vi "UV Laser Ablation and Capture.vi"() -> ()   [LabVIEW 2016]
uses:
  <vilib>/vision/NI_Vision_Development_Module.lvlib
  C:/Users/Murray group/Desktop/LabVIEW Version Controlled/UV Laser Ablation Capture Software/uc480DotNet.dll
  uc480DotNet.dll
  System.Windows.Forms
  <vilib>/Utility/miscctls.llb/LVBoundsTypeDef.ctl
  <vilib>/Utility/config.llb/NI_LVConfig.lvlib
  <vilib>/regexp/Match Regular Expression.xnode
panel:
  in  "Load ROI":bool
  in  "Save current ROI":bool
  in  "Call Last ROI":bool
  in  "Captur time\nConstant":dbl=0.001 min=0.001 step=0.001 format="%#_13g"
  out "Pre-Capture Axis 2":dbl format="%.10e"
  out "Pre-Capture Axis 1":dbl format="%.10e"
  in  "Log files":bool
  out "Axis 2 inverted?":bool
  out "Axis 1 inverted?":bool
  out "Rect height\n(px)":i32
  out "Rect width\n(px)":i32
  in  "Circle?":bool=TRUE
  out "Axis 2 group":i32
  out "Axis 1 group":i32
  in  "Microscope/Capture \nstatus button":bool=TRUE
  in  "X travel":dbl min=0.0 max=150.0 step=0.0001
  in  "Y travel":dbl min=0.0 max=150.0 step=0.0001
  in  "Laser Status":bool
  in  "SINGLE SHOT":bool
  in  "Repetition\nRate (Hz)":dbl=2.34 min=1.0 max=20.0 step=0.01 format="%.2g"
  out "Laser Com Delay":i32
  out "VISA Laser port":string
  in  "Acceleration \n(mm/s²)":dbl=20.0
  out "Camera Status":string="Load parameter"
  in  "Save configuration":bool
  in  "Stages status":bool
  in  "Transparency":u8 max=80 step=1
  in  "Overlay MSI Image":bool
  in  "Home Axes":bool
  out "Axis 2 Offset":dbl
  out "Axis 1 Offset":dbl
  out "Acceleration":dbl
  out "Velocity":dbl
  in  "Axis Initial Parameters":T1={"Velocity (units/seconds)"=1.0, "Acceleration (units/seconds²)"=20.0, "Minimum Jerk Time (seconds)"=0.005, "Maximum Jerk Time (seconds)"=0.009} {"Maximum Jerk Time (seconds)" format="%.6e"; "Minimum Jerk Time (seconds)" format="%.6e"; "Acceleration (units/seconds²)" format="%.6e"; "Velocity (units/seconds)" format="%.6e"}
  out "Axis 2":string
  out "Axis 1":string
  out "XPS_Address":string
  in  "Axes Manual Control":bool
  out "ROI Area \n(mm2)":dbl=4.035870075999999
  out "Laser on/off array":bool[][](array[boolean])
  out "Commands array":string[][](array[string])
  in  "Exit Camera":bool
  in  "Width (px)":i32=240
  in  "X offset":i32=406 step=1
  in  "Y offset":i32=693 step=1
  out "Processi time (sec)":i32=117
  in  "Processing time unit":string(combo)="sec"
  out "Process time":dbl=117.0
  in  "Mode":i32(ring) items=["RGB 32"=0, "RGB 24"=1, "Y8 Monochrom"=6]
  in  "Camera":refnum<k24>(container)
  in  "Init Camera":bool
  in  "Start Live":bool
  in  "Stop Live":bool
  in  "Load Parameter":bool
  out "Error Out":errorcluster caption="error"
  out "Bits/Pixel":i32=32
  out "Width":i32=1280
  out "Height":i32=1024
  out "Serial Number":string="4102944807"
  in  "Camera ID":i32
  in  "Zoom":dbl(ring)=1.5 items=["4X"=4.0, "2X"=2.0, "1.5X"=1.5, "1.25X"=1.25, "1X"=1.0]
  in  "Gain Boost":bool=TRUE
  in  "Snapshot":bool
  out "Output":picture
  in  "Exposure":dbl(slide)=99.80425000000001 min=0.06241666666666667 max=99.80425000000001 step=0.06241666666666667 scale=0.06241666666666667..99.80425000000001 scale format="%#.3g"
  in  "Framerate":dbl(slide)=10.002522802986672 min=0.47411700449083627 max=15.001275108384213 step=0.014032998230481021 scale=0.47411700449083627..15.001275108384213 scale format="%#.3g"
  in  "Pixelclock":i32(slide)=24 min=5 max=40 step=1 scale=5.0..40.0
  in  "error in (no error)":errorcluster
  out "error out":errorcluster
  in  "Precision (%)":dbl=1.0 min=1.0 max=100.0 step=1.0 format="%#_3g"
  in  "Process Image":bool
  in  "Pixel size":dbl=12.19 step=0.01
  in  "Speed (µm/s)":i32=1000
  in  "Heigth (px)":i32=240
  in  "Height \nstep divider":i32=2
  out "Rect height\n(µm/px)":i32=2267
  out "Rect. width \n(µm/px))":i32=2267
  out "Source":T2(plugin-control)
  in  "Open \nManual":bool
  in  "Capture":bool
  out "Log":string
  out "Laser Operation":bool
  in  "LASER":bool
  in  "LAMP":bool
  in  "EXIT":bool
  # "Laser Control"
  # "Stages Control"
  # "Camera Control"
  # "ROI Processing"
  # "Laser spot size and position"
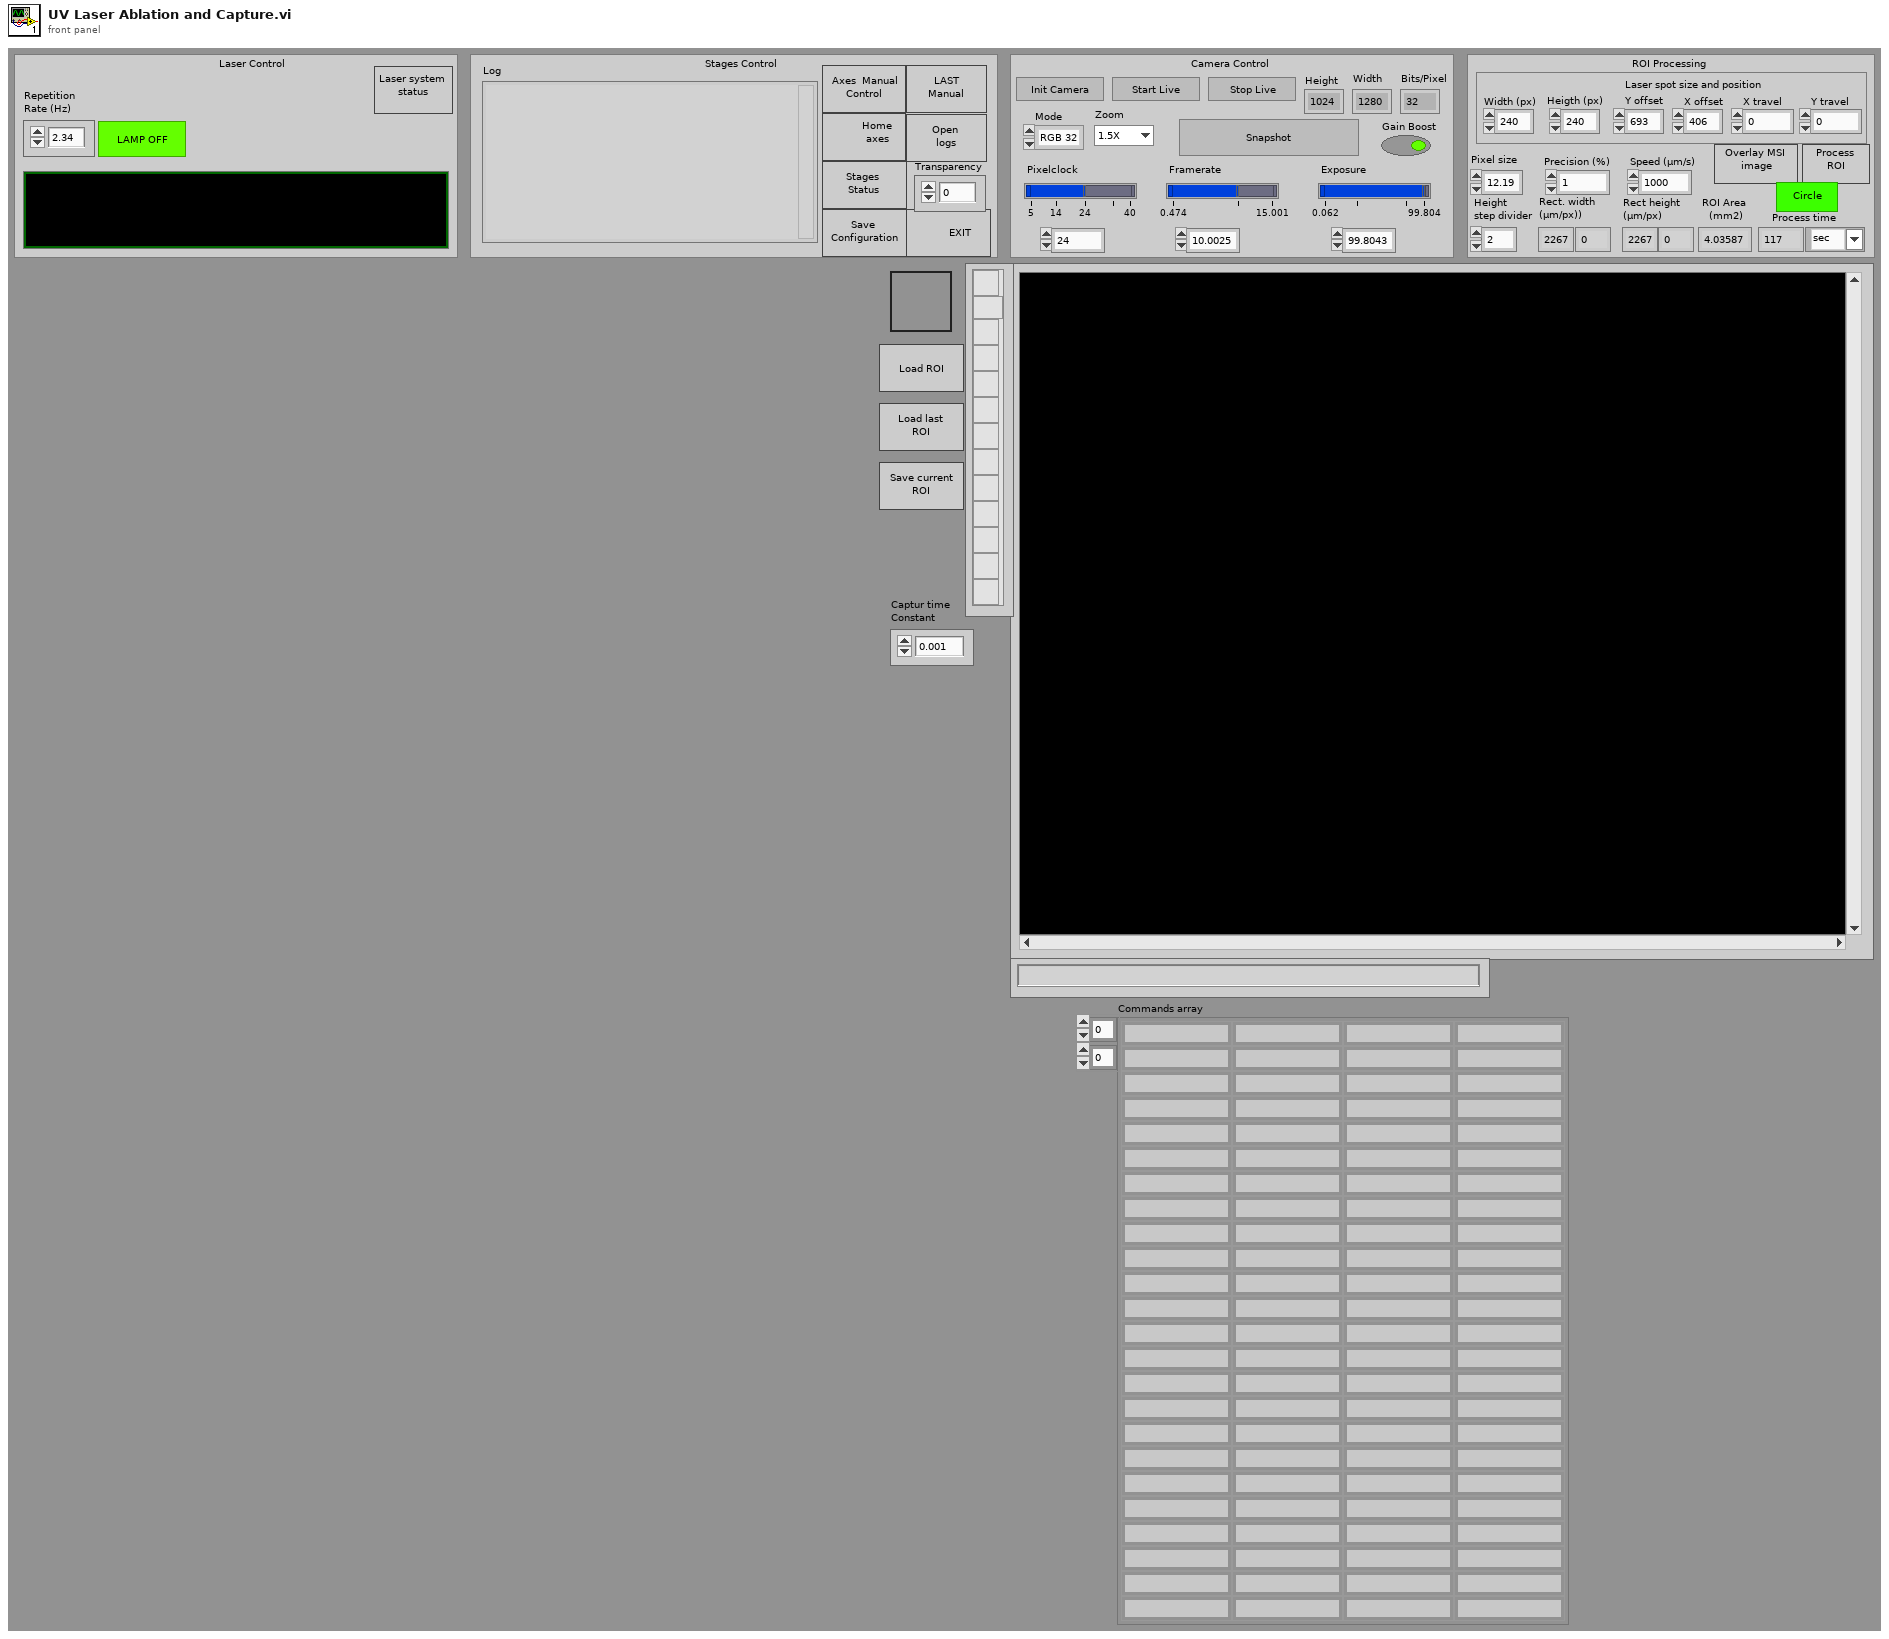
[diagram p1: front panel]
types:
  T1 = cluster{"Velocity (units/seconds)":dbl, "Acceleration (units/seconds²)":dbl, "Minimum Jerk Time (seconds)":dbl, "Maximum Jerk Time (seconds)":dbl}
  T2 = typedef "IMAQ Image.ctl" = refnum<image>
  T3 = typedef "LVBoundsTypeDef.ctl" = cluster{"Width":u32, "Height":u32}
  T4 = enum8{"Enabled", "Disabled", "Disabled and Grayed Out"}
  T5 = typedef "NI_LVConfig.lvlib/Config Data RefNum.ctl" = refnum<k1>
  T6 = enum16{"open", "replace", "create", "open or create", "replace or create", "replace or create with confirmation"}
  T7 = enum32{"Invalid", "Standard", "Closed", "Hidden", "Minimized", "Maximized"}
  T8 = enum32{"invalid app kind", "Development System", "Run Time System", "Student Edition", "Embedded LabVIEW", "Evaluation", "Custom"}
  T9 = cluster{"connection TCP":refnum<k5>, "LogTo File":bool, "Log File refnum":refnum<file>, "no error if error log":bool}
  T10 = typedef "Image Type" = u32
  T11 = cluster{"Global Rectangle":i32[], "Contours":cluster{"Contour Type":u32, "ROI Type":u32, "Points":i32[]}[]}
  T12 = cluster{"Global Rectangle[0]":i32, "Global Rectangle[1]":i32}
  T13 = typedef "ROI Descriptor" = cluster{"Global Rectangle":i32[], "Contours":cluster{"ID":enum32{"External", "Internal"}, "Type":u32, "Coordinates":i32[]}[]}
  T14 = cluster{"ID":enum32{"External", "Internal"}, "Type":u32, "Coordinates":i32[]}[]
  T15 = cluster{"ID":enum32{"External", "Internal"}, "Type":u32, "Coordinates":i32[]}
  T16 = cluster{"Contour Type":u32, "ROI Type":u32, "Points":i32[]}[]
  T17 = cluster{"Contour Type":u32, "ROI Type":u32, "Points":i32[]}
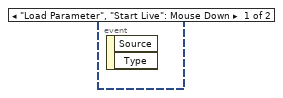
[diagram p2: hidden frame]
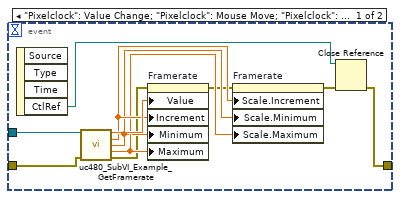
[diagram p3: hidden frame]
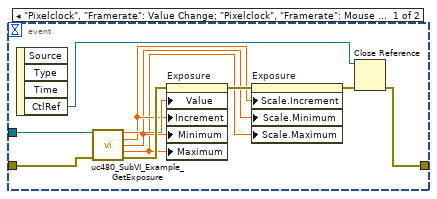
[diagram p4: hidden frame]
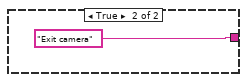
[diagram p5: hidden frame]
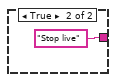
[diagram p6: hidden frame]
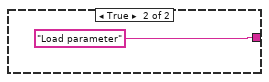
[diagram p7: hidden frame]
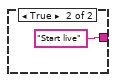
[diagram p8: hidden frame]
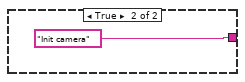
[diagram p9: hidden frame]
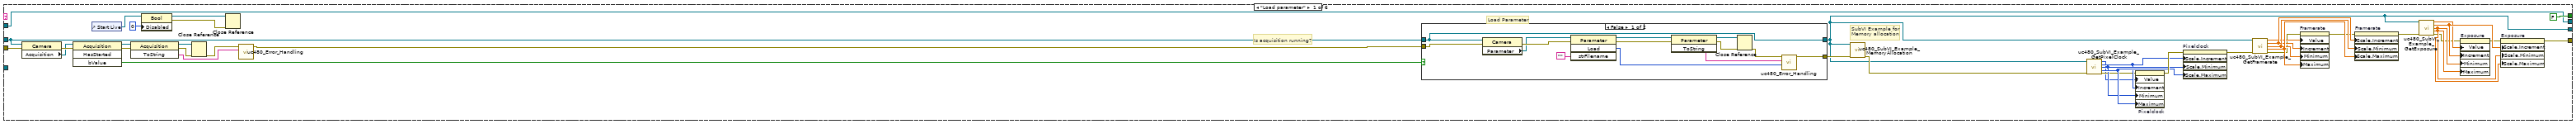
[diagram p10: hidden frame]
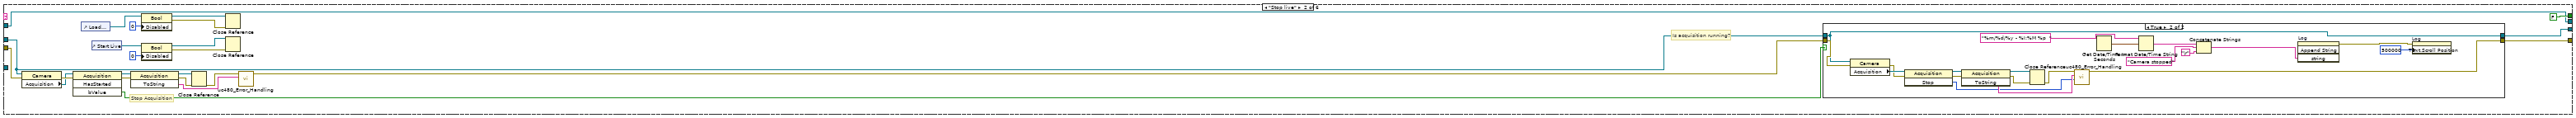
[diagram p12: hidden frame]
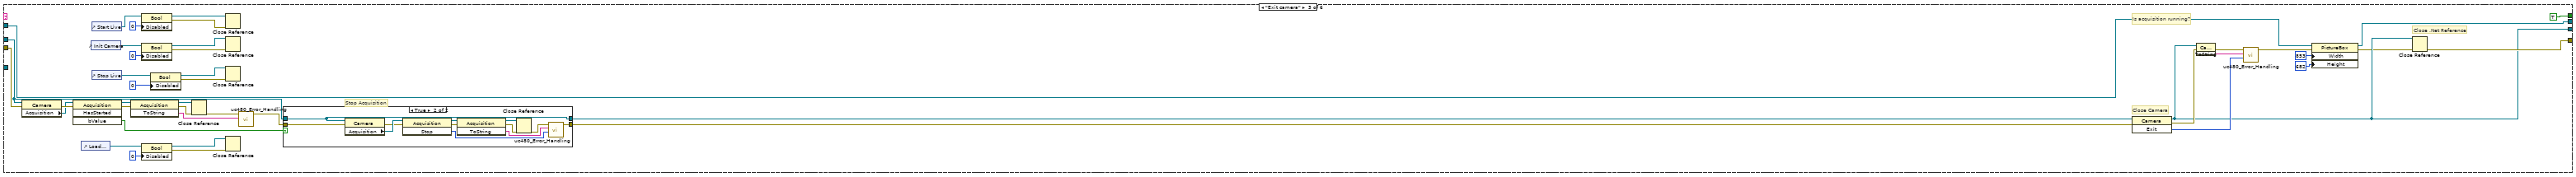
[diagram p14: hidden frame]
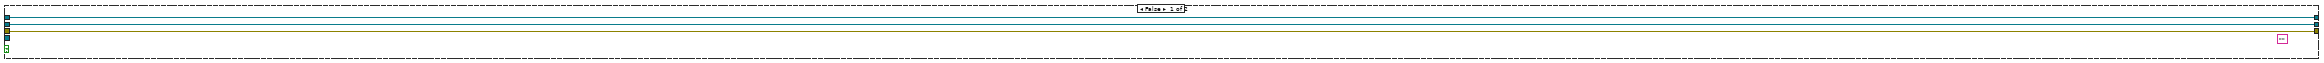
[diagram p16: hidden frame]
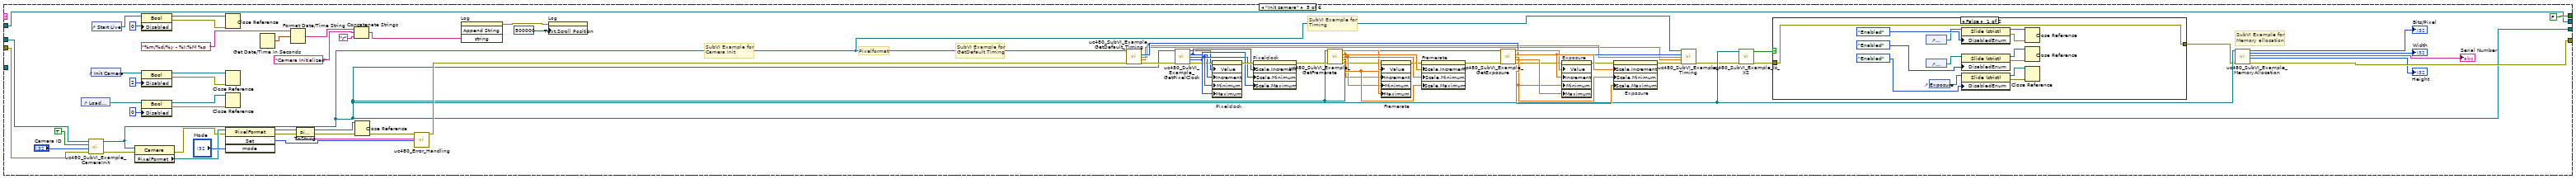
[diagram p18: hidden frame]
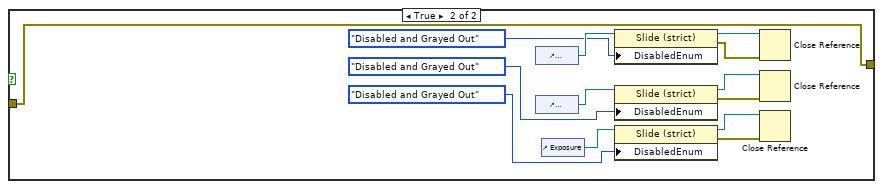
[diagram p19: hidden frame]
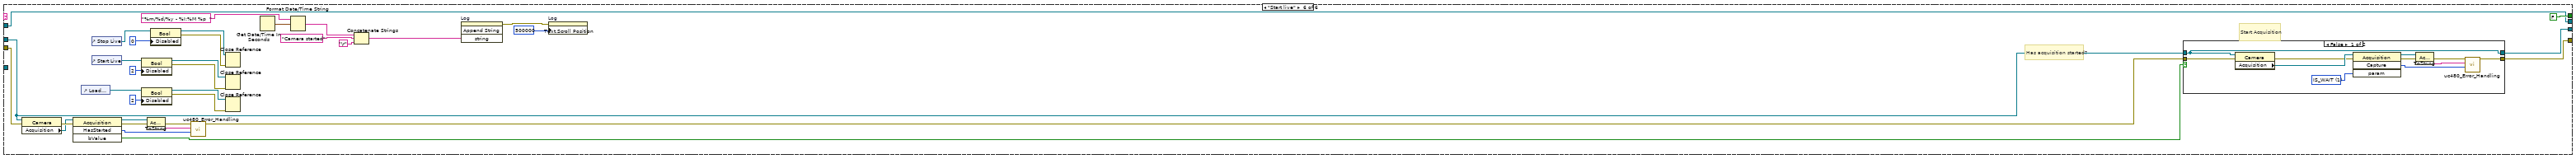
[diagram p20: hidden frame]
diagram:
  w65 = 1 items=["None", "FixedSingle", "Fixed3D"] ("BorderStyle")
  # "Button and controls"
  # "Camera control buttons"
  n1 = property class="PictureBox"(reference="Camera", "BorderStyle"=w65, "Width"=853, "Height"=682) -> (reference out=w53:refnum<k24>, error out=w54:errorcluster)  [unwired: 1 in]
  n2 = property class="PictureBox"(reference=w53, error in=w54) -> (reference out=w52:refnum<k24>, error out=w51:errorcluster, "Handle"=w50:refnum<k24>)
  n3 = while "Camera Control" {
    shift-right: [w82] -> _
    shift-left: w51 -> [w88]
    shift-right: [w85] -> _
    shift-left: _ -> [w78]
    shift-right: [w80] -> _
    shift-left: w52 -> [w81]
    tunnel: w50 -> [w79]
    stop <- w86 stop-if-true
    # ".NetReference"
    # ".Net Reference"
    n4 = event shown="[1] Timeout" {
      selector: _ -> [_ _]
      dyn-events: _ -> [_ _]
      timeout: 0 -> [_ _]
      event "Load Parameter", "Start Live": Mouse Down {
        n5 = event-data() -> ()  [unwired: 1 in, 2 out]
      }
      event Timeout {
        n6 = event-data() -> ()  [unwired: 1 in, 2 out]
      }
    }
    n7 = event shown="[1] Timeout" {
      selector: _ -> [_ _]
      dyn-events: _ -> [_ _]
      timeout: 0 -> [_ _]
      tunnel: [w102 w113] -> w89
      tunnel: w88 -> [w112 w113]
      tunnel: w78 -> [w111 _]
      event "Pixelclock": Value Change; "Pixelclock": Mouse Move; "Pixelclock": Key Down; "Pixelclock": Mouse Up {
        n8 = event-data() -> ("CtlRef"=w104:refnum<vi>)  [unwired: 1 in, 3 out]
        n9 = call "uc480_SubVI_Example_GetFramerate.vi"(".NET (Reference)"=w111, "Error In"=w112) -> ("Framerate"=w110:dbl, "Inc"=w109:dbl, "Min"=w107:dbl, "Max"=w108:dbl, "error out"=w106:errorcluster)  [unwired: 9 in]
        n10 = property on="Framerate" class="Slide (strict)"(error in=w106, "Value"=w110, "Increment"=w109, "Minimum"=w107, "Maximum"=w108) -> (error out=w105:errorcluster)  [unwired: 1 in, 1 out]
        n11 = property on="Framerate" class="Slide (strict)"(error in=w105, "Scale.Increment"=w109, "Scale.Minimum"=w107, "Scale.Maximum"=w108) -> (error out=w103:errorcluster)  [unwired: 1 in, 1 out]
        n12 = Close Reference(reference=w104, error in (no error)=w103) -> (error out=w102:errorcluster)
      }
      event Timeout {
        n13 = event-data() -> ()  [unwired: 1 in, 2 out]
      }
    }
    n14 = case shown="False" "Load Parameter" {
      tunnel: ["" "Load parameter"] -> w95
      frame False {
      }
      frame True {
      }
    }
    n15 = case shown="False" "Init Camera" {
      tunnel: ["" "Init camera"] -> w99
      frame False {
      }
      frame True {
      }
    }
    n16 = case shown="False" "Exit Camera" {
      tunnel: ["" "Exit camera"] -> w93
      frame False {
      }
      frame True {
      }
    }
    n17 = event shown="[1] Timeout" {
      selector: _ -> [_ _]
      dyn-events: _ -> [_ _]
      timeout: 0 -> [_ _]
      tunnel: w89 -> [w124 w125]
      tunnel: [w114 w125] -> w91
      tunnel: w78 -> [w123 _]
      event "Pixelclock", "Framerate": Value Change; "Pixelclock", "Framerate": Mouse Move; "Pixelclock", "Framerate": Key Down; "Pixelclock", "Framerate": Mouse Up {
        n18 = event-data() -> ("CtlRef"=w116:refnum<vi>)  [unwired: 1 in, 3 out]
        n19 = call "uc480_SubVI_Example_GetExposure.vi"(".NET (Reference)"=w123, "Error In"=w124) -> ("Exposure"=w120:dbl, "Inc"=w119:dbl, "Min"=w118:dbl, "Max"=w117:dbl, "Error out"=w121:errorcluster)  [unwired: 9 in]
        n20 = property on="Exposure" class="Slide (strict)"(error in=w121, "Value"=w120, "Increment"=w119, "Minimum"=w118, "Maximum"=w117) -> (error out=w122:errorcluster)  [unwired: 1 in, 1 out]
        n21 = property on="Exposure" class="Slide (strict)"(error in=w122, "Scale.Increment"=w119, "Scale.Minimum"=w118, "Scale.Maximum"=w117) -> (error out=w115:errorcluster)  [unwired: 1 in, 1 out]
        n22 = Close Reference(reference=w116, error in (no error)=w115) -> (error out=w114:errorcluster)
      }
      event Timeout {
        n23 = event-data() -> ()  [unwired: 1 in, 2 out]
      }
    }
    n24 = case shown="False" "Start Live" {
      tunnel: ["" "Start live"] -> w98
      frame False {
      }
      frame True {
      }
    }
    n25 = case shown="False" "Stop Live" {
      tunnel: ["" "Stop live"] -> w94
      frame False {
      }
      frame True {
      }
    }
    n26 = local read "Camera Status"() -> (w75:string)
    n27 = Concatenate Strings(w99, w98, w95, w94, w93) -> (→"Camera Status":string)
    n28 = case shown="Default" w75 {
      tunnel: w78 -> [w168 w208 w266 w308 w488 w547]
      tunnel: w91 -> [w171 w209 w267 w318 w487 w548]
      tunnel: [w142 w207 w275 w317 w446 w546] -> w85
      tunnel: [w143 w206 w276 w316 w483 w544] -> w84
      tunnel: [FALSE FALSE TRUE FALSE FALSE FALSE] -> w86
      tunnel: w81 -> [w141 w200 w248 w300 w441 w537]
      tunnel: [w141 w200 w247 w299 w441 w537] -> w80
      tunnel: w79 -> [_ _ _ w296 _ _]
      frame "Load parameter" {
        # "SubVI Example for \nMemory allocation"
        # "Is acquisition running?"
        # "Load Parameter"
        n29 = property class="Camera"(reference=w168, error in=w171) -> (error out=w176:errorcluster, "Acquisition"=w175:refnum<k24>)  [unwired: 1 out]
        n30 = invoke class="Acquisition" method="HasStarted"(reference=w175, error in=w176) -> (reference out=w172:refnum<k24>, error out=w174:errorcluster, "bValue"=w170:bool)  [unwired: 2 in, 1 out]
        n31 = control-ref of="Start Live"() -> (w166:refnum<vi>)
        n32 = invoke class="Acquisition" method="ToString"(reference=w172, error in=w174) -> (reference out=w138:refnum<k24>, error out=w137:errorcluster, "ToString"=w173:string)  [unwired: 1 in]
        n33 = property class="Bool"(reference=w166, "Disabled"=u8 0 ("Deaktiviert")) -> (reference out=w140:refnum<vi>, error out=w139:errorcluster)  [unwired: 1 in]
        n34 = Close Reference(reference=w138, error in (no error)=w137) -> (error out=w136:errorcluster)
        n35 = Close Reference(reference=w140, error in (no error)=w139) -> ()  [unwired: 1 out]
        n36 = call "uc480_Error_Handling.vi"("Error String"=w173, "Error In"=w136) -> ("Error Out"=w169:errorcluster)  [unwired: 9 in]
        n37 = case shown="False" w170 {
          tunnel: w169 -> [w184 w191]
          tunnel: w168 -> [w182 w192]
          tunnel: [w183 w191] -> w167
          tunnel: [w182 w192] -> w142
          frame False {
            n38 = property class="Camera"(reference=w182, error in=w184) -> (error out=w186:errorcluster, "Parameter"=w185:refnum<k24>)  [unwired: 1 out]
            n39 = invoke class="Parameter" method="Load"(reference=w185, error in=w186, "strFilename"="") -> (reference out=w188:refnum<k24>, error out=w189:errorcluster, "Load"=w181:i32)  [unwired: 1 in, 1 out]
            n40 = invoke class="Parameter" method="ToString"(reference=w188, error in=w189) -> (reference out=w178:refnum<k24>, error out=w180:errorcluster, "ToString"=w190:string)  [unwired: 1 in]
            n41 = Close Reference(reference=w178, error in (no error)=w180) -> (error out=w179:errorcluster)
            n42 = call "uc480_Error_Handling.vi"("Error Code"=w181, "Error String"=w190, "Error In"=w179) -> ("Error Out"=w183:errorcluster)  [unwired: 8 in]
          }
          frame True {
          }
        }
        n43 = call "uc480_SubVI_Example_MemoryAllocation.vi"(".NET (Reference)"=w142, "Error In"=w167) -> ("Error Out"=w144:errorcluster)  [unwired: 13 in, 4 out]
        n44 = call "uc480_SubVI_Example_GetPixelClock.vi"(".NET (Reference)"=w142, "Error In"=w144) -> ("Pixel Clock"=w145:i32, "Inc"=w147:i32, "Min"=w148:i32, "Max"=w149:i32, "error out"=w146:errorcluster)  [unwired: 9 in]
        n45 = property on="Pixelclock" class="Slide (strict)"(error in=w146, "Value"=w145, "Increment"=w147, "Minimum"=w148, "Maximum"=w149) -> (error out=w150:errorcluster)  [unwired: 1 in, 1 out]
        n46 = property on="Pixelclock" class="Slide (strict)"(error in=w150, "Scale.Increment"=w147, "Scale.Minimum"=w148, "Scale.Maximum"=w149) -> (error out=w151:errorcluster)  [unwired: 1 in, 1 out]
        n47 = call "uc480_SubVI_Example_GetFramerate.vi"(".NET (Reference)"=w142, "Error In"=w151) -> ("Framerate"=w154:dbl, "Inc"=w155:dbl, "Min"=w156:dbl, "Max"=w157:dbl, "error out"=w153:errorcluster)  [unwired: 9 in]
        n48 = property on="Framerate" class="Slide (strict)"(error in=w153, "Value"=w154, "Increment"=w155, "Minimum"=w156, "Maximum"=w157) -> (error out=w152:errorcluster)  [unwired: 1 in, 1 out]
        n49 = property on="Framerate" class="Slide (strict)"(error in=w152, "Scale.Increment"=w155, "Scale.Minimum"=w156, "Scale.Maximum"=w157) -> (error out=w158:errorcluster)  [unwired: 1 in, 1 out]
        n50 = call "uc480_SubVI_Example_GetExposure.vi"(".NET (Reference)"=w142, "Error In"=w158) -> ("Exposure"=w161:dbl, "Inc"=w162:dbl, "Min"=w163:dbl, "Max"=w164:dbl, "Error out"=w159:errorcluster)  [unwired: 9 in]
        n51 = property on="Exposure" class="Slide (strict)"(error in=w159, "Value"=w161, "Increment"=w162, "Minimum"=w163, "Maximum"=w164) -> (error out=w160:errorcluster)  [unwired: 1 in, 1 out]
        n52 = property on="Exposure" class="Slide (strict)"(error in=w160, "Scale.Increment"=w162, "Scale.Minimum"=w163, "Scale.Maximum"=w164) -> (error out=w143:errorcluster)  [unwired: 1 in, 1 out]
      }
      frame "Stop live" {
        # "Is acquisition running?"
        # "Stop Acquisition"
        n53 = property class="Camera"(reference=w208, error in=w209) -> (error out=w216:errorcluster, "Acquisition"=w215:refnum<k24>)  [unwired: 1 out]
        n54 = invoke class="Acquisition" method="HasStarted"(reference=w215, error in=w216) -> (reference out=w210:refnum<k24>, error out=w212:errorcluster, "bValue"=w214:bool)  [unwired: 2 in, 1 out]
        n55 = control-ref of="Load Parameter"() -> (w204:refnum<vi>)
        n56 = control-ref of="Start Live"() -> (w201:refnum<vi>)
        n57 = invoke class="Acquisition" method="ToString"(reference=w210, error in=w212) -> (reference out=w193:refnum<k24>, error out=w195:errorcluster, "ToString"=w211:string)  [unwired: 1 in]
        n58 = property class="Bool"(reference=w204, "Disabled"=u8 0 ("Deaktiviert")) -> (reference out=w199:refnum<vi>, error out=w198:errorcluster)  [unwired: 1 in]
        n59 = property class="Bool"(reference=w201, "Disabled"=u8 0 ("Deaktiviert")) -> (reference out=w197:refnum<vi>, error out=w196:errorcluster)  [unwired: 1 in]
        n60 = Close Reference(reference=w193, error in (no error)=w195) -> (error out=w194:errorcluster)
        n61 = Close Reference(reference=w199, error in (no error)=w198) -> ()  [unwired: 1 out]
        n62 = Close Reference(reference=w197, error in (no error)=w196) -> ()  [unwired: 1 out]
        n63 = call "uc480_Error_Handling.vi"("Error String"=w211, "Error In"=w194) -> ("Error Out"=w213:errorcluster)  [unwired: 9 in]
        n64 = case shown="True" w214 {
          tunnel: [w218 w237] -> w206
          tunnel: w213 -> [w218 w238]
          tunnel: w208 -> [w217 w230]
          tunnel: [w217 w230] -> w207
          frame False {
          }
          frame True {
            n65 = property class="Camera"(reference=w230, error in=w238) -> (error out=w234:errorcluster, "Acquisition"=w235:refnum<k24>)  [unwired: 1 out]
            n66 = invoke class="Acquisition" method="Stop"(reference=w235, error in=w234) -> (reference out=w232:refnum<k24>, error out=w233:errorcluster, "Stop"=w231:i32)  [unwired: 1 in]
            n67 = invoke class="Acquisition" method="ToString"(reference=w232, error in=w233) -> (reference out=w227:refnum<k24>, error out=w229:errorcluster, "ToString"=w236:string)  [unwired: 1 in]
            n68 = Close Reference(reference=w227, error in (no error)=w229) -> (error out=w228:errorcluster)
            n69 = call "uc480_Error_Handling.vi"("Error Code"=w231, "Error String"=w236, "Error In"=w228) -> ("Error Out"=w237:errorcluster)  [unwired: 8 in]
            n70 = Get Date/Time In Seconds() -> (seconds since 1Jan1904=w225:timestamp)
            n71 = Format Date/Time String(time format string (%c)="%m/%d/%y - %I:%M %p  ", seconds (now)=w225) -> (date/time string=w226:string)  [unwired: 1 in]
            n72 = Concatenate Strings(w226, "Camera stopped", "\r") -> (w221:string)
            n73 = invoke on="Log" class="Str" method="Append String"("string"=w221) -> (error out=w219:errorcluster)  [unwired: 3 in, 3 out]
            n74 = property on="Log" class="Str"(error in=w219, "Text.Scroll Position"=u32 500000) -> ()  [unwired: 1 in, 2 out]
          }
        }
      }
      frame "Exit camera" {
        # "Close .Net Reference"
        # "Is acquisition running?"
        # "Stop Acquisition"
        # "Close Camera"
        n75 = property class="Camera"(reference=w266, error in=w267) -> (error out=w274:errorcluster, "Acquisition"=w273:refnum<k24>)  [unwired: 1 out]
        n76 = invoke class="Acquisition" method="HasStarted"(reference=w273, error in=w274) -> (reference out=w268:refnum<k24>, error out=w270:errorcluster, "bValue"=w272:bool)  [unwired: 2 in, 1 out]
        n77 = control-ref of="Load Parameter"() -> (w257:refnum<vi>)
        n78 = control-ref of="Init Camera"() -> (w259:refnum<vi>)
        n79 = control-ref of="Start Live"() -> (w258:refnum<vi>)
        n80 = control-ref of="Stop Live"() -> (w256:refnum<vi>)
        n81 = invoke class="Acquisition" method="ToString"(reference=w268, error in=w270) -> (reference out=w253:refnum<k24>, error out=w255:errorcluster, "ToString"=w269:string)  [unwired: 1 in]
        n82 = property class="Bool"(reference=w258, "Disabled"=u8 0 ("Deaktiviert")) -> (reference out=w242:refnum<vi>, error out=w241:errorcluster)  [unwired: 1 in]
        n83 = property class="Bool"(reference=w259, "Disabled"=u8 0 ("Deaktiviert")) -> (reference out=w240:refnum<vi>, error out=w239:errorcluster)  [unwired: 1 in]
        n84 = property class="Bool"(reference=w257, "Disabled"=u8 0 ("Deaktiviert")) -> (reference out=w244:refnum<vi>, error out=w243:errorcluster)  [unwired: 1 in]
        n85 = property class="Bool"(reference=w256, "Disabled"=u8 0 ("Deaktiviert")) -> (reference out=w246:refnum<vi>, error out=w245:errorcluster)  [unwired: 1 in]
        n86 = Close Reference ("Close Referenz")(reference=w253, error in (no error)=w255) -> (error out=w254:errorcluster)
        n87 = Close Reference(reference=w242, error in (no error)=w241) -> ()  [unwired: 1 out]
        n88 = Close Reference(reference=w240, error in (no error)=w239) -> ()  [unwired: 1 out]
        n89 = Close Reference(reference=w246, error in (no error)=w245) -> ()  [unwired: 1 out]
        n90 = Close Reference(reference=w244, error in (no error)=w243) -> ()  [unwired: 1 out]
        n91 = call "uc480_Error_Handling.vi"("Error String"=w269, "Error In"=w254) -> ("Error Out"=w271:errorcluster)  [unwired: 9 in]
        n92 = case shown="True" w272 {
          tunnel: [w283 w294] -> w264
          tunnel: w271 -> [w283 w295]
          tunnel: w266 -> [w282 w287]
          tunnel: [w282 w287] -> w265
          frame False {
          }
          frame True {
            n93 = property class="Camera"(reference=w287, error in=w295) -> (error out=w291:errorcluster, "Acquisition"=w292:refnum<k24>)  [unwired: 1 out]
            n94 = invoke class="Acquisition" method="Stop"(reference=w292, error in=w291) -> (reference out=w289:refnum<k24>, error out=w290:errorcluster, "Stop"=w288:i32)  [unwired: 1 in]
            n95 = invoke class="Acquisition" method="ToString"(reference=w289, error in=w290) -> (reference out=w284:refnum<k24>, error out=w286:errorcluster, "ToString"=w293:string)  [unwired: 1 in]
            n96 = Close Reference ("Close Referenz")(reference=w284, error in (no error)=w286) -> (error out=w285:errorcluster)
            n97 = call "uc480_Error_Handling.vi"("Error Code"=w288, "Error String"=w293, "Error In"=w285) -> ("Error Out"=w294:errorcluster)  [unwired: 8 in]
          }
        }
        n98 = invoke class="Camera" method="Exit"(reference=w265, error in=w264) -> (reference out=w275:refnum<k24>, error out=w278:errorcluster, "Exit"=w277:i32)  [unwired: 1 in]
        n99 = invoke class="Camera" method="ToString"(reference=w275, error in=w278) -> (error out=w279:errorcluster, "ToString"=w280:string)  [unwired: 1 in, 1 out]
        n100 = call "uc480_Error_Handling.vi"("Error Code"=w277, "Error String"=w280, "Error In"=w279) -> ("Error Out"=w252:errorcluster)  [unwired: 8 in]
        n101 = property class="PictureBox"(reference=w248, error in=w252, "Width"=853, "Height"=682) -> (reference out=w247:refnum<k24>, error out=w251:errorcluster)
        n102 = Close Reference ("Close Referenz")(reference=w275, error in (no error)=w251) -> (error out=w276:errorcluster)
      }
      frame Default {
        # "SubVI Example for Timing"
        # "Has acquisition started?"
        n103 = call "uc480_SubVI_Example_Timing.vi"(".NET (Reference)"=w308, "Pixelclock"="Pixelclock", "Exposure time"="Exposure", "Framerate"="Framerate", "Error In"=w318) -> ("Pixelclock"=w311:i32, "Exposure time"=w310:dbl, "Framerate"=w309:dbl, "Error Out"=w315:errorcluster)  [unwired: 7 in]
        n104 = property on="Framerate" class="Schieber (strikt)"(error in=w315, "Scale.RngStart"=w309) -> (error out=w314:errorcluster)  [unwired: 1 in, 1 out]
        n105 = property on="Exposure" class="Schieber (strikt)"(error in=w314, "Scale.RngStart"=w310) -> (error out=w313:errorcluster)  [unwired: 1 in, 1 out]
        n106 = property on="Pixelclock" class="Schieber (strikt)"(error in=w313, "Scale.RngStart"=w311) -> (error out=w312:errorcluster)  [unwired: 1 in, 1 out]
        n107 = property class="Camera"(reference=w308, error in=w312) -> (reference out=w301:refnum<k24>, error out=w324:errorcluster, "Acquisition"=w323:refnum<k24>)
        n108 = invoke class="Acquisition" method="HasStarted"(reference=w323, error in=w324) -> (reference out=w298:refnum<k24>, error out=w320:errorcluster, "HasStarted"=w319:i32, "bValue"=w297:bool)  [unwired: 2 in]
        n109 = invoke class="Acquisition" method="ToString"(reference=w298, error in=w320) -> (reference out=w302:refnum<k24>, error out=w322:errorcluster, "ToString"=w321:string)  [unwired: 1 in]
        n110 = call "uc480_Error_Handling.vi"("Error Code"=w319, "Error String"=w321, "Error In"=w322) -> ("Error Out"=w304:errorcluster)  [unwired: 8 in]
        n111 = Close Reference(reference=w302, error in (no error)=w304) -> (error out=w303:errorcluster)
        n112 = case "Show Image" shown="True" w297 {
          tunnel: [w328 w340] -> w316
          tunnel: w303 -> [w328 w368]
          tunnel: w301 -> [w327 w332]
          tunnel: [w327 w336] -> w317
          tunnel: w300 -> [w326 w357]
          tunnel: [w326 w334] -> w299
          tunnel: w296 -> [_ w364]
          frame False {
            (unwired) ""
          }
          frame True {
            n113 = local read "Height"() -> (w361:i32)
            n114 = local read "Width"() -> (w362:i32)
            n115 = Quotient & Remainder(x=w362, y="Zoom") -> (floor(x/y)=w359:dbl)  [unwired: 1 out]
            n116 = Quotient & Remainder(x=w361, y="Zoom") -> (floor(x/y)=w358:dbl)  [unwired: 1 out]
            n117 = To Long Integer(number=w359) -> (32bit integer=w331:i32)
            n118 = To Long Integer(number=w358) -> (32bit integer=w330:i32)
            n119 = property class="PictureBox"(reference=w357, error in=w368, "Width"=w331, "Height"=w330) -> (reference out=w334:refnum<k24>, error out=w363:errorcluster)
            n120 = property class="Camera"(reference=w332, error in=w363) -> (reference out=w333:refnum<k24>, error out=w370:errorcluster, "Memory"=w371:refnum<k24>)
            n121 = invoke class="Memory" method="GetActive"(reference=w371, error in=w370) -> (reference out=w365:refnum<k24>, error out=w366:errorcluster, "s32MemId"=w337:i32)  [unwired: 2 in, 1 out]
            n122 = property class="Camera"(reference=w333, error in=w366) -> (reference out=w345:refnum<k24>, error out=w369:errorcluster, "Display"=w354:refnum<k24>)
            n123 = invoke class="Display" method="Render"(reference=w354, error in=w369, "memID"=w337, "windowHandle"=w364) -> (reference out=w355:refnum<k24>, error out=w356:errorcluster)  [unwired: 1 in, 3 out]
            n124 = property class="Camera"(reference=w345, error in=w356) -> (reference out=w336:refnum<k24>, error out=w352:errorcluster, "Gain"=w350:refnum<k24>)
            n125 = property class="Gain"(reference=w350, error in=w352) -> (reference out=w351:refnum<k24>, error out=w347:errorcluster, "Hardware"=w346:refnum<k24>)
            n126 = property class="GainHardware"(reference=w346, error in=w347) -> (reference out=w343:refnum<k24>, error out=w348:errorcluster, "Boost"=w349:refnum<k24>)
            n127 = property class="GainBoost"(reference=w349, error in=w348, "Enabled"="Gain Boost") -> (reference out=w344:refnum<k24>, error out=w335:errorcluster)
            n128 = case "Snapshot control" shown="True" "Snapshot" {
              tunnel: w332 -> [_ w392]
              tunnel: w335 -> [w372 w396]
              tunnel: [w372 w383] -> w329
              tunnel: w331 -> [_ w386]
              tunnel: w330 -> [_ w385]
              frame False {
              }
              frame True {
                n129 = property class="Camera"(reference=w392, error in=w396) -> (error out=w416:errorcluster, "Memory"=w415:refnum<k24>)  [unwired: 1 out]
                n130 = local read "Zoom"() -> (w391:dbl)
                n131 = invoke class="Memory" method="GetList"(reference=w415, error in=w416) -> (reference out=w421:refnum<k24>, error out=w420:errorcluster, "GetList"=w422:i32, "idList"=w409:i32[])  [unwired: 2 in]
                n132 = Bundle(cluster=T3 {"Width"=0, "Height"=0} ("Draw Area Size"), "Width"=w386, "Height"=w385) -> (w387:T3)
                n133 = Divide(x=1.0, y=w391) -> (x/y=w389:dbl)
                n134 = property on="Output" class="Pict"("ZoomFactor"=w389, "Draw Area Size"=w387) -> ()  [unwired: 2 in, 2 out]
                n135 = invoke class="Memory" method="ToString"(reference=w421, error in=w420) -> (reference out=w394:refnum<k24>, error out=w404:errorcluster, "ToString"=w419:string)  [unwired: 1 in]
                n136 = Index Array(array=w409, index=0 ("Active \nAcquisition Buffer")) -> (element=w406:i32)
                n137 = Index Array(array=w409, index=u32 0 ("Active \nOutput Buffer")) -> (element=w405:i32)
                n138 = Close Reference(reference=w394, error in (no error)=w404) -> (error out=w403:errorcluster)
                n139 = call "uc480_Error_Handling.vi"("Error Code"=w422, "Error String"=w419, "Error In"=w403) -> ("Error Out"=w412:errorcluster)  [unwired: 8 in]
                n140 = Get Date/Time In Seconds() -> (seconds since 1Jan1904=w376:timestamp)
                n141 = property class="Camera"(reference=w392, error in=w412) -> (error out=w411:errorcluster, "Memory"=w410:refnum<k24>)  [unwired: 1 out]
                n142 = Format Date/Time String(time format string (%c)="%m/%d/%y -%I:%M %p  ", seconds (now)=w376) -> (date/time string=w375:string)  [unwired: 1 in]
                n143 = invoke class="Memory" method="SetActive"(reference=w410, error in=w411, "s32MemId"=w406) -> (reference out=w395:refnum<k24>, error out=w402:errorcluster)  [unwired: 1 in, 2 out]
                n144 = Concatenate Strings(w375, "Snapshot taken", "\r") -> (w380:string)
                n145 = Close Reference(reference=w395, error in (no error)=w402) -> (error out=w401:errorcluster)
                n146 = invoke on="Log" class="Str" method="Append String"("string"=w380) -> (error out=w373:errorcluster)  [unwired: 3 in, 3 out]
                n147 = property class="Camera"(reference=w392, error in=w401) -> (error out=w418:errorcluster, "Memory"=w407:refnum<k24>)  [unwired: 1 out]
                n148 = invoke class="Memory" method="CopyToArray"(reference=w407, error in=w418, "s32MemId"=w405) -> (reference out=w397:refnum<k24>, error out=w398:errorcluster, "u8Image"=w417:u8[])  [unwired: 2 in, 2 out]
                n149 = property on="Log" class="Str"(error in=w373, "Text.Scroll Position"=u32 500000) -> ()  [unwired: 1 in, 2 out]
                n150 = invoke class="Memory" method="ToString"(reference=w397, error in=w398) -> (reference out=w393:refnum<k24>, error out=w400:errorcluster, "ToString"=w423:string)  [unwired: 1 in]
                n151 = Close Reference(reference=w393, error in (no error)=w400) -> (error out=w399:errorcluster)
                n152 = call "uc480_Error_Handling.vi"("Error String"=w423, "Error In"=w399) -> ("Error Out"=w414:errorcluster)  [unwired: 9 in]
                n153 = call "uc480_ArrayToImage.vi"("Error In"=w414, "InArray"=w417, ".NET (Reference)"=w392) -> ("Error Out"=w382:errorcluster, "Image"=w384:picture)  [unwired: 7 in]
                "Output" <- w384
                n154 = call "Picture to IMAQ.vi"("Error In"=w382, "picture"=w384) -> ("Error Out"=w383:errorcluster, "Image"=→"Source":T2)  [unwired: 8 in]
              }
            }
            n155 = Close Reference(reference=w343, error in (no error)=w329) -> (error out=w342:errorcluster)
            n156 = Close Reference(reference=w344, error in (no error)=w342) -> (error out=w339:errorcluster)
            n157 = Close Reference(reference=w351, error in (no error)=w339) -> (error out=w353:errorcluster)
            n158 = Close Reference(reference=w355, error in (no error)=w353) -> (error out=w367:errorcluster)
            n159 = Close Reference(reference=w365, error in (no error)=w367) -> (error out=w340:errorcluster)
          }
        }
      }
      frame "Init camera" {
        # "SubVI Example for \nGetDefault Timing"
        # "SubVI Example for \nMemory allocation"
        # "SubVI Example for \nTiming"
        # "SubVI Example for \nCamera Init"
        # "Pixelformat"
        n160 = control-ref of="Load Parameter"() -> (w447:refnum<vi>)
        n161 = call "uc480_SubVI_Example_CameraInit.vi"("Error In"=w487, "Camera ID"="Camera ID", "Init Camera Flag"=TRUE, ".NET (Reference)"=w488) -> ("Error Out"=w493:errorcluster, ".NET (Reference)"=w446:refnum<k24>)  [unwired: 6 in]
        n162 = control-ref of="Init Camera"() -> (w451:refnum<vi>)
        n163 = control-ref of="Start Live"() -> (w449:refnum<vi>)
        n164 = property on="Property Node" class="Camera"(reference=w446, error in=w493) -> (error out=w494:errorcluster, "PixelFormat"=w495:refnum<k24>)  [unwired: 1 out]
        n165 = property class="Bool"(reference=w449, "Disabled"=u8 0 ("Deaktiviert")) -> (reference out=w438:refnum<vi>, error out=w437:errorcluster)  [unwired: 1 in]
        n166 = property class="Bool"(reference=w451, "Disabled"=u8 2 ("Deaktiviert")) -> (reference out=w440:refnum<vi>, error out=w439:errorcluster)  [unwired: 1 in]
        n167 = property class="Bool"(reference=w447, "Disabled"=u8 0 ("Deaktiviert")) -> (reference out=w436:refnum<vi>, error out=w435:errorcluster)  [unwired: 1 in]
        n168 = Close Reference(reference=w438, error in (no error)=w437) -> ()  [unwired: 1 out]
        n169 = Close Reference(reference=w440, error in (no error)=w439) -> ()  [unwired: 1 out]
        n170 = Close Reference(reference=w436, error in (no error)=w435) -> ()  [unwired: 1 out]
        n171 = invoke class="PixelFormat" method="Set"(reference=w495, error in=w494, "mode"="Mode") -> (reference out=w491:refnum<k24>, error out=w484:errorcluster, "Set"=w490:i32)  [unwired: 1 in, 1 out]
        n172 = Get Date/Time In Seconds() -> (seconds since 1Jan1904=w427:timestamp)
        n173 = Format Date/Time String(time format string (%c)="%m/%d/%y - %I:%M %p  ", seconds (now)=w427) -> (date/time string=w426:string)  [unwired: 1 in]
        n174 = invoke class="PixelFormat" method="ToString"(reference=w491, error in=w484) -> (reference out=w432:refnum<k24>, error out=w434:errorcluster, "ToString"=w492:string)  [unwired: 1 in]
        n175 = Concatenate Strings(w426, "Camera Initialized", "\r") -> (w431:string)
        n176 = Close Reference(reference=w432, error in (no error)=w434) -> (error out=w433:errorcluster)
        n177 = call "uc480_Error_Handling.vi"("Error Code"=w490, "Error String"=w492, "Error In"=w433) -> ("Error Out"=w458:errorcluster)  [unwired: 8 in]
        n178 = invoke on="Log" class="Str" method="Append String"("string"=w431) -> (error out=w424:errorcluster)  [unwired: 3 in, 3 out]
        n179 = property on="Log" class="Str"(error in=w424, "Text.Scroll Position"=u32 500000) -> ()  [unwired: 1 in, 2 out]
        n180 = call "uc480_SubVI_Example_GetDefault_Timing.vi"(".NET (Reference)"=w446, "Error In"=w458) -> ("Pixelclock"=w457:i32, "Exposure time"=w456:dbl, "Framerate"=w455:dbl, "Error Out"=w454:errorcluster)  [unwired: 10 in]
        n181 = call "uc480_SubVI_Example_GetPixelClock.vi"(".NET (Reference)"=w446, "Error In"=w454) -> ("Pixel Clock"=w459:i32, "Inc"=w461:i32, "Min"=w462:i32, "Max"=w463:i32, "error out"=w460:errorcluster)  [unwired: 9 in]
        n182 = property on="Pixelclock" class="Slide (strict)"(error in=w460, "Value"=w459, "Increment"=w461, "Minimum"=w462, "Maximum"=w463) -> (error out=w464:errorcluster)  [unwired: 1 in, 1 out]
        n183 = property on="Pixelclock" class="Slide (strict)"(error in=w464, "Scale.Increment"=w461, "Scale.Minimum"=w462, "Scale.Maximum"=w463) -> (error out=w465:errorcluster)  [unwired: 1 in, 1 out]
        n184 = call "uc480_SubVI_Example_GetFramerate.vi"(".NET (Reference)"=w446, "Error In"=w465) -> ("Framerate"=w468:dbl, "Inc"=w469:dbl, "Min"=w470:dbl, "Max"=w471:dbl, "error out"=w467:errorcluster)  [unwired: 9 in]
        n185 = property on="Framerate" class="Slide (strict)"(error in=w467, "Value"=w468, "Increment"=w469, "Minimum"=w470, "Maximum"=w471) -> (error out=w466:errorcluster)  [unwired: 1 in, 1 out]
        n186 = property on="Framerate" class="Slide (strict)"(error in=w466, "Scale.Increment"=w469, "Scale.Minimum"=w470, "Scale.Maximum"=w471) -> (error out=w472:errorcluster)  [unwired: 1 in, 1 out]
        n187 = call "uc480_SubVI_Example_GetExposure.vi"(".NET (Reference)"=w446, "Error In"=w472) -> ("Exposure"=w475:dbl, "Inc"=w476:dbl, "Min"=w477:dbl, "Max"=w478:dbl, "Error out"=w473:errorcluster)  [unwired: 9 in]
        n188 = property on="Exposure" class="Slide (strict)"(error in=w473, "Value"=w475, "Increment"=w476, "Minimum"=w477, "Maximum"=w478) -> (error out=w474:errorcluster)  [unwired: 1 in, 1 out]
        n189 = property on="Exposure" class="Slide (strict)"(error in=w474, "Scale.Increment"=w476, "Scale.Minimum"=w477, "Scale.Maximum"=w478) -> (error out=w453:errorcluster)  [unwired: 1 in, 1 out]
        n190 = call "uc480_SubVI_Example_Timing.vi"(".NET (Reference)"=w446, "Pixelclock"=w457, "Exposure time"=w456, "Framerate"=w455, "Error In"=w453) -> ("Error Out"=w445:errorcluster)  [unwired: 7 in, 3 out]
        n191 = call "uc480_SubVI_Example_Is_XS.vi"("Error In"=w445, ".NET (Reference)"=w446) -> ("Error Out"=w442:errorcluster, "IsXS"=w444:bool)  [unwired: 7 in, 1 out]
        n192 = case shown="False" w444 {
          tunnel: w442 -> [w509 w522]
          tunnel: [w509 w522] -> w443
          frame False {
            n193 = control-ref of="Pixelclock"() -> (w505:refnum<vi>)
            n194 = control-ref of="Framerate"() -> (w504:refnum<vi>)
            n195 = control-ref of="Exposure"() -> (w503:refnum<vi>)
            n196 = property class="Slide (strict)"(reference=w505, "DisabledEnum"=T4."Enabled" ("Disabled")) -> (reference out=w502:refnum<vi>, error out=w501:errorcluster)  [unwired: 1 in]
            n197 = property class="Slide (strict)"(reference=w504, "DisabledEnum"=T4."Enabled" ("Disabled")) -> (reference out=w500:refnum<vi>, error out=w499:errorcluster)  [unwired: 1 in]
            n198 = property class="Slide (strict)"(reference=w503, "DisabledEnum"=T4."Enabled" ("Disabled")) -> (reference out=w498:refnum<vi>, error out=w497:errorcluster)  [unwired: 1 in]
            n199 = Close Reference(reference=w502, error in (no error)=w501) -> ()  [unwired: 1 out]
            n200 = Close Reference(reference=w500, error in (no error)=w499) -> ()  [unwired: 1 out]
            n201 = Close Reference(reference=w498, error in (no error)=w497) -> ()  [unwired: 1 out]
          }
          frame True {
            n202 = control-ref of="Pixelclock"() -> (w521:refnum<vi>)
            n203 = control-ref of="Framerate"() -> (w518:refnum<vi>)
            n204 = control-ref of="Exposure"() -> (w516:refnum<vi>)
            n205 = property class="Slide (strict)"(reference=w521, "DisabledEnum"=T4."Disabled and Grayed Out" ("Disabled")) -> (reference out=w514:refnum<vi>, error out=w515:errorcluster)  [unwired: 1 in]
            n206 = property class="Slide (strict)"(reference=w518, "DisabledEnum"=T4."Disabled and Grayed Out" ("Disabled")) -> (reference out=w513:refnum<vi>, error out=w512:errorcluster)  [unwired: 1 in]
            n207 = property class="Slide (strict)"(reference=w516, "DisabledEnum"=T4."Disabled and Grayed Out" ("Disabled")) -> (reference out=w511:refnum<vi>, error out=w510:errorcluster)  [unwired: 1 in]
            n208 = Close Reference(reference=w514, error in (no error)=w515) -> ()  [unwired: 1 out]
            n209 = Close Reference(reference=w513, error in (no error)=w512) -> ()  [unwired: 1 out]
            n210 = Close Reference(reference=w511, error in (no error)=w510) -> ()  [unwired: 1 out]
          }
        }
        n211 = call "uc480_SubVI_Example_MemoryAllocation.vi"(".NET (Reference)"=w446, "Error In"=w443) -> ("Bits/Pixel 2"=→"Bits/Pixel":i32, "Width"=→"Width":i32, "Serial Number"=→"Serial Number":string, "Height"=→"Height":i32, "Error Out"=w483:errorcluster)  [unwired: 13 in]
      }
      frame "Start live" {
        # "Has acquisition started?"
        # "Start Acquisition"
        n212 = property class="Camera"(reference=w547, error in=w548) -> (error out=w557:errorcluster, "Acquisition"=w556:refnum<k24>)  [unwired: 1 out]
        n213 = invoke class="Acquisition" method="HasStarted"(reference=w556, error in=w557) -> (reference out=w552:refnum<k24>, error out=w551:errorcluster, "HasStarted"=w550:i32, "bValue"=w555:bool)  [unwired: 2 in]
        n214 = control-ref of="Load Parameter"() -> (w540:refnum<vi>)
        n215 = control-ref of="Stop Live"() -> (w538:refnum<vi>)
        n216 = control-ref of="Start Live"() -> (w543:refnum<vi>)
        n217 = property class="Bool"(reference=w543, "Disabled"=u8 2 ("Deaktiviert")) -> (reference out=w532:refnum<vi>, error out=w531:errorcluster)  [unwired: 1 in]
        n218 = property class="Bool"(reference=w540, "Disabled"=u8 2 ("Deaktiviert")) -> (reference out=w534:refnum<vi>, error out=w533:errorcluster)  [unwired: 1 in]
        n219 = invoke class="Acquisition" method="ToString"(reference=w552, error in=w551) -> (error out=w554:errorcluster, "ToString"=w553:string)  [unwired: 1 in, 1 out]
        n220 = property class="Bool"(reference=w538, "Disabled"=u8 0 ("Deaktiviert")) -> (reference out=w536:refnum<vi>, error out=w535:errorcluster)  [unwired: 1 in]
        n221 = call "uc480_Error_Handling.vi"("Error Code"=w550, "Error String"=w553, "Error In"=w554) -> ("Error Out"=w549:errorcluster)  [unwired: 8 in]
        n222 = Close Reference(reference=w536, error in (no error)=w535) -> ()  [unwired: 1 out]
        n223 = Close Reference(reference=w532, error in (no error)=w531) -> ()  [unwired: 1 out]
        n224 = Close Reference(reference=w534, error in (no error)=w533) -> ()  [unwired: 1 out]
        n225 = Get Date/Time In Seconds() -> (seconds since 1Jan1904=w526:timestamp)
        n226 = Format Date/Time String(time format string (%c)="%m/%d/%y - %I:%M %p  ", seconds (now)=w526) -> (date/time string=w525:string)  [unwired: 1 in]
        n227 = Concatenate Strings(w525, "Camera started", "\r") -> (w530:string)
        n228 = invoke on="Log" class="Str" method="Append String"("string"=w530) -> (error out=w523:errorcluster)  [unwired: 3 in, 3 out]
        n229 = property on="Log" class="Str"(error in=w523, "Text.Scroll Position"=u32 500000) -> ()  [unwired: 1 in, 2 out]
        n230 = case shown="False" w555 {
          tunnel: [w560 w570] -> w544
          tunnel: w549 -> [w566 w570]
          tunnel: w547 -> [w565 w569]
          tunnel: [w565 w569] -> w546
          frame False {
            w558 = 1 items=["IS_DONT_WAIT", "IS_WAIT"] ("Wait")
            n231 = property class="Camera"(reference=w565, error in=w566) -> (error out=w567:errorcluster, "Acquisition"=w568:refnum<k24>)  [unwired: 1 out]
            n232 = invoke class="Acquisition" method="Capture"(reference=w568, error in=w567, "param"=w558) -> (reference out=w561:refnum<k24>, error out=w562:errorcluster, "Capture"=w559:i32)  [unwired: 1 in, 1 out]
            n233 = invoke class="Acquisition" method="ToString"(reference=w561, error in=w562) -> (error out=w564:errorcluster, "ToString"=w563:string)  [unwired: 1 in, 1 out]
            n234 = call "uc480_Error_Handling.vi"("Error Code"=w559, "Error String"=w563, "Error In"=w564) -> ("Error Out"=w560:errorcluster)  [unwired: 8 in]
          }
          frame True {
          }
        }
      }
    }
    n235 = call "uc480_SubVI_Example_SyncEventLoop.vi"("Error In"=w84, "use sync"=w86, ".NET (Reference)"=w85) -> ("Error Out"=w82:errorcluster, "Synchronize (ms)"=w83:dbl)  [unwired: 7 in]
    "Error Out" <- w82
    n236 = Wait Until Next ms Multiple(millisecond multiple=w83) -> ()  [unwired: 1 out]
  }
  n237 = flat-sequence "Initialization sequence" {
    tunnel: [w597] -> w38
    tunnel: [w581] -> w36
    tunnel: [w580] -> w35
    tunnel: [w577] -> w33
    tunnel: [w576] -> w32
    tunnel: [w573] -> w21
    tunnel: [w572] -> w2
    tunnel: [w571] -> w1
    tunnel: w38 -> [w739]
    tunnel: [w733] -> w37
    tunnel: w36 -> [w732]
    tunnel: w35 -> [w731]
    tunnel: [w730] -> w34
    tunnel: w33 -> [w730]
    tunnel: w32 -> [w729]
    tunnel: [w729] -> w31
    tunnel: [w728] -> w22
    tunnel: w21 -> [w728]
    tunnel: [w727] -> w10
    tunnel: [w726] -> w6
    tunnel: w2 -> [w727]
    tunnel: w1 -> [w726]
    tunnel: [w754] -> w49
    tunnel: [w745] -> w48
    tunnel: [w746] -> w44
    tunnel: w37 -> [w750]
    tunnel: w34 -> [w744]
    tunnel: w31 -> [w743]
    tunnel: [w742] -> w23
    tunnel: w22 -> [w742]
    tunnel: w10 -> [w741]
    tunnel: [w741] -> w9
    tunnel: w6 -> [w740]
    tunnel: [w740] -> w5
    tunnel: w49 -> [w760]
    tunnel: [w760] -> w47
    tunnel: w48 -> [w759]
    tunnel: [w758] -> w45
    tunnel: w44 -> [w758]
    tunnel: [w757] -> w30
    tunnel: w23 -> [w757]
    tunnel: w9 -> [w756]
    tunnel: [w756] -> w8
    tunnel: w5 -> [w755]
    tunnel: [w755] -> w4
    tunnel: w47 -> [w767]
    tunnel: [w767] -> w46
    tunnel: w45 -> [w766]
    tunnel: w30 -> [w765]
    tunnel: [w765] -> w29
    tunnel: w8 -> [w764]
    tunnel: [w764] -> w7
    tunnel: w4 -> [w763]
    tunnel: [w763] -> w3
    tunnel: [w777] -> w43
    tunnel: w46 -> [w777]
    tunnel: w29 -> [w772]
    tunnel: [w772] -> w28
    tunnel: [w771] -> w20
    tunnel: [w770] -> w15
    tunnel: w7 -> [w771]
    tunnel: w3 -> [w770]
    tunnel: w43 -> [w782]
    tunnel: [w782] -> w42
    tunnel: w28 -> [w780]
    tunnel: [w780] -> w27
    tunnel: w20 -> [w779]
    tunnel: [w779] -> w19
    tunnel: w15 -> [w778]
    tunnel: [w778] -> w14
    tunnel: w42 -> [w787]
    tunnel: [w787] -> w41
    tunnel: w27 -> [w785]
    tunnel: [w785] -> w26
    tunnel: w19 -> [w784]
    tunnel: [w784] -> w18
    tunnel: w14 -> [w783]
    tunnel: [w783] -> w13
    tunnel: w41 -> [w792]
    tunnel: [w792] -> w40
    tunnel: w26 -> [w790]
    tunnel: [w790] -> w25
    tunnel: w18 -> [w789]
    tunnel: [w789] -> w17
    tunnel: w13 -> [w788]
    tunnel: [w788] -> w12
    tunnel: w40 -> [w797]
    tunnel: [w797] -> w39
    tunnel: w25 -> [w795]
    tunnel: [w795] -> w24
    tunnel: w17 -> [w794]
    tunnel: [w794] -> w16
    tunnel: w12 -> [w793]
    tunnel: [w793] -> w11
    tunnel: w39 -> [w801]
    tunnel: w24 -> [w800]
    tunnel: w16 -> [w799]
    tunnel: w11 -> [w798]
    frame #0 {
      w598 = "standby" ("regular expression")
      w608 = FALSE ("Visible")
      n238 = control-ref of="This VI"() -> (w609:refnum<vi>)
      n239 = control-ref of="This VI"() -> (w607:refnum<vi>)
      n240 = invoke class="VI" method="Default Vals.Reinit All"(reference=w609) -> ()  [unwired: 2 in, 3 out]
      n241 = property on="Axes Manual Control" class="Bool (strict)"("Visible"=w608) -> ()  [unwired: 2 in, 2 out]
      n242 = property on="Home Axes" class="Bool"("Visible"=w608) -> ()  [unwired: 2 in, 2 out]
      n243 = property class="VI"(reference=w607) -> ("Path"=w606:path)  [unwired: 1 in, 2 out]
      n244 = Strip Path(path=w606) -> (stripped path=w605:path)  [unwired: 1 out]
      n245 = Build Path(base path=w605, name or relative path="General_Configuration.ini") -> (appended path=w603:path)
      n246 = call <vilib>:"Open Config Data.vi"("create file if necessary (T)"=FALSE, "configuration file path"=w603) -> ("error out"=w578:errorcluster, "refnum"=w579:T5)  [unwired: 7 in, 1 out]
      n247 = call "Configuration reader.vi"("refnum"=w579, "error in (no error)"=w578) -> ("Velocity"=→"Velocity":dbl, "Exposure"=w572:dbl, "X offset"=w590:i32, "Y travel"=w588:dbl, "X travel"=w587:dbl, "Y offset"=w589:i32, "Acceleration"=→"Acceleration":dbl, "Pixelclock"=w573:i32, "Framerate"=w571:dbl, "Width (px)"=w592:i32, "Speed (µm/s)"=w596:i32, "XPS_Address"=→"XPS_Address":string, "Axis 1 group"=w577:i32, "Precision (%)"=w593:dbl, "Pixel size"=w594:dbl, "Axis 2 inverted?"=→"Axis 2 inverted?":bool, "Axis 1 inverted?"=→"Axis 1 inverted?":bool, "Heigth (px)"=w591:i32, "Laser Com Delay"=w580:i32, "Height  step \ndivider"=w595:i32, "VISA Laser port"=w581:string, "Axis 2 group"=w576:i32, "error out"=w583:errorcluster)  [unwired: 3 in]
      "VISA Laser port" <- w581
      "Laser Com Delay" <- w580
      "Axis 1 group" <- w577
      "Axis 2 group" <- w576
      n248 = local write "Heigth (px)"(w591) -> ()
      n249 = local write "Pixel size"(w594) -> ()
      n250 = local write "Precision (%)"(w593) -> ()
      n251 = local write "Speed (µm/s)"(w596) -> ()
      n252 = local write "Width (px)"(w592) -> ()
      n253 = local write "Y offset"(w590) -> ()
      n254 = local write "X travel"(w587) -> ()
      n255 = local write "X offset"(w589) -> ()
      n256 = local write "Y travel"(w588) -> ()
      n257 = local write "Height \nstep divider"(w595) -> ()
      n258 = call "CheckStatus.vi"("Error In"=w583, "delay before read (ms)"=w580, "VISA resource name"=w581) -> ("Error Out"=w582:errorcluster, "read buffer"=w601:string)  [unwired: 5 in, 2 out]
      n259 = xnode "Match Regular Expression"("input string"=w601, "regular expression"=w598, "error in"=w582) -> ("whole match"=w599:string, "error out"=w597:errorcluster)  [unwired: 3 in, 3 out]
      n260 = Equal?(x=w599, y=w598) -> (x = y?=w600:bool)
      n261 = case shown="True" w600 {
        frame False {
        }
        frame True {
          n262 = control-ref of="Log"() -> (w725:refnum<vi>)
          n263 = call "Log writer.vi"("reference"=w725, "string"="Initializing the ICE450 Ultra..." ("Initialiazation")) -> ()  [unwired: 10 in]
        }
      }
    }
    frame #1 {
      n264 = call "ICE450 Ultra Initialization.vi"("error in (no error)"=w739, "delay before read (ms)"=w731, "VISA resource name"=w732) -> ("Error Out"=w733:errorcluster, "Repetition rate"=w734:dbl, "Laser initialization status"=w738:string)  [unwired: 6 in]
      n265 = local write "Repetition\nRate (Hz)"(w734) -> ()
      n266 = property on="Log" class="Str"("Text.Scroll Position"=u32 500000) -> ()  [unwired: 2 in, 2 out]
      n267 = Concatenate Strings(w738, "\r") -> (w736:string)
      n268 = invoke on="Log" class="Str" method="Append String"("string"=w736) -> ()  [unwired: 3 in, 4 out]
    }
    frame #2 {
      n269 = local read "XPS_Address"() -> (w747:string)
      n270 = control-ref of="Log"() -> (w748:refnum<vi>)
      n271 = call "Axes initialization.vi"("Axis 2 group"=w743, "Axis 1 group"=w744, "error in (no error)"=w750, "Axis Initial Parameters"="Axis Initial Parameters", "reference"=w748, "XPS_Address"=w747) -> ("Error out"=w751:errorcluster, "Axis 1"=→"Axis 1":string, "Axis 1 ready?"=w745:bool, "Axis 2"=→"Axis 2":string, "Axes 2 ready?"=w746:bool)
      n272 = call <vilib>:"Simple Error Handler.vi"("error in (no error)"=w751) -> ()  [unwired: 4 in, 5 out]
      n273 = And(x=w745, y=w746) -> (x .and. y?=w754:bool)
    }
    frame #3 {
      n274 = case shown="True" w759 {
        frame False {
        }
        frame True {
          n275 = control-ref of="Log"() -> (w762:refnum<vi>)
          n276 = call "Log writer.vi"("reference"=w762, "string"="Axis 1 ready" ("Initialiazation")) -> ()  [unwired: 10 in]
        }
      }
    }
    frame #4 {
      n277 = case shown="True" w766 {
        frame False {
        }
        frame True {
          n278 = control-ref of="Log"() -> (w768:refnum<vi>)
          n279 = call "Log writer.vi"("reference"=w768, "string"="Axis 2 ready" ("Initialiazation")) -> ()  [unwired: 10 in]
        }
      }
    }
    frame #5 {
      w773 = FALSE ("Visible")
      # "Set defaults"
      n280 = property on="LAMP" class="Bool (strict)"("BoolText.Text"="LAMP OFF" ("Boolean Text.Text")) -> ()  [unwired: 2 in, 2 out]
      n281 = property on="Laser Operation" class="Bool (strict)"("Blinking"=w773) -> ()  [unwired: 2 in, 2 out]
      n282 = property on="Capture" class="Bool"("Visible"=w773) -> ()  [unwired: 2 in, 2 out]
      n283 = property on="SINGLE SHOT" class="Bool"("Visible"=w773) -> ()  [unwired: 2 in, 2 out]
      n284 = property on="LASER" class="Bool (strict)"("BoolText.Text"="LASER OFF" ("Boolean Text.Text"), "Visible"=FALSE) -> ()  [unwired: 2 in, 2 out]
    }
    frame #6 {
      n285 = local write "Camera Status"("Init camera" ("Camera Status")) -> ()
    }
    frame #7 {
      n286 = Wait (ms)(milliseconds to wait=u32 1000) -> ()  [unwired: 1 out]
    }
    frame #8 {
      n287 = local write "Camera Status"("Start live") -> ()
    }
    frame #9 {
      n288 = Wait (ms)(milliseconds to wait=u32 1000) -> ()  [unwired: 1 out]
    }
    frame #10 {
      n289 = case shown="True" w801 {
        frame False {
          n290 = One Button Dialog(message="Axes not ready") -> ()  [unwired: 1 in, 1 out]
        }
        frame True {
          n291 = property on="Axes Manual Control" class="Bool (strict)"("Visible"=TRUE) -> ()  [unwired: 2 in, 2 out]
          n292 = property on="Home Axes" class="Bool"("Visible"=TRUE) -> ()  [unwired: 2 in, 2 out]
          n293 = control-ref of="Log"() -> (w804:refnum<vi>)
          n294 = call "Log writer.vi"("reference"=w804, "string"="System ready" ("Initialiazation")) -> ()  [unwired: 10 in]
        }
      }
      n295 = local write "Framerate"(w798) -> ()
      n296 = local write "Pixelclock"(w800) -> ()
      n297 = local write "Exposure"(w799) -> ()
    }
  }
  n298 = while "Laser control & Stages Control" {
    stop <- w819 stop-if-true
    n299 = local read "Laser Com Delay"() -> (w807:i32)
    n300 = local read "VISA Laser port"() -> (w808:string)
    n301 = local read "XPS_Address"() -> (w811:string)
    n302 = local read "Axis 2"() -> (w809:string)
    n303 = local read "Axis 1"() -> (w810:string)
    n304 = event shown="[12] \"Process Image\": Value Change" {
      selector: _ -> [_ _ _ _ _ _ _ _ _ _ _ _ _ _ _ _ _ _ _ _ _]
      dyn-events: _ -> [_ _ _ _ _ _ _ _ _ _ _ _ _ _ _ _ _ _ _ _ _]
      timeout: _ -> [_ _ _ _ _ _ _ _ _ _ _ _ _ _ _ _ _ _ _ _ _]
      tunnel: [_ _ _ w1151 _ _ _ _ _ _ _ _ _ _ _ _ _ _ _ _ _] -> w819
      tunnel: [w826 w982 w1145 _ _ _ _ w1212 _ w1240 w1267 _ w1331 _ _ _ "" ("StringOut") w1603 _ w1727 w1880] -> w812
      tunnel: w811 -> [_ _ _ _ _ _ _ _ _ _ w1270 _ _ _ _ _ w1520 w1602 _ w1714 w1871]
      tunnel: w810 -> [_ _ _ _ _ _ _ _ _ _ w1269 _ _ _ _ _ w1519 w1601 _ w1713 w1881]
      tunnel: w809 -> [_ _ _ _ _ _ _ _ _ _ w1268 _ _ _ _ _ w1518 w1600 _ w1712 w1882]
      tunnel: w808 -> [w824 w980 w1142 w1150 _ _ _ w1215 w1235 _ _ _ _ _ _ _ _ _ _ _ _]
      tunnel: w807 -> [w823 w979 w1141 w1149 _ _ _ w1214 w1234 _ _ _ _ _ _ _ _ _ _ _ _]
      event "LAMP": Value Change {
        n305 = event-data() -> ()  [unwired: 1 in, 6 out]
        n306 = case shown="True" "LAMP" {
          tunnel: [w827 w955] -> w826
          tunnel: w824 -> [w833 w954]
          tunnel: w823 -> [w832 w953]
          frame False {
            w828 = "standby" ("regular expression")
            n307 = call "FLStop.vi"("delay before read (ms)"=w832, "VISA resource name"=w833) -> ("read buffer"=w831:string)  [unwired: 6 in, 3 out]
            n308 = xnode "Match Regular Expression"("input string"=w831, "regular expression"=w828) -> ("whole match"=w829:string)  [unwired: 4 in, 4 out]
            n309 = Equal?(x=w829, y=w828) -> (x = y?=w830:bool)
            n310 = case shown="True" w830 {
              tunnel: ["" "Flashlamp deactivated"] -> w827
              frame False {
              }
              frame True {
                w835 = FALSE ("Visible")
                n311 = property on="LASER" class="Bool (strict)"("Visible"=w835) -> ()  [unwired: 2 in, 2 out]
                n312 = property on="Capture" class="Bool"("Visible"=w835) -> ()  [unwired: 2 in, 2 out]
                n313 = property on="SINGLE SHOT" class="Bool"("Visible"=w835) -> ()  [unwired: 2 in, 2 out]
                n314 = property on="Laser Operation" class="Bool (strict)"("Blinking"=w835) -> ()  [unwired: 2 in, 2 out]
                n315 = property on="LAMP" class="Bool (strict)"("BoolText.Text"="LAMP OFF" ("Boolean Text.Text")) -> ()  [unwired: 2 in, 2 out]
              }
            }
          }
          frame True {
            n316 = flat-sequence {
              tunnel: w954 -> [w963]
              tunnel: w953 -> [w962]
              tunnel: [w959] -> w952
              tunnel: [w973] -> w955
              tunnel: w952 -> [w972]
              frame #0 {
                w960 = "fire" ("regular expression")
                n317 = while {
                  i -> [w967]
                  stop <- w970 stop-if-true
                  n318 = Wait Until Next ms Multiple(millisecond multiple=u32 1000) -> ()  [unwired: 1 out]
                  n319 = Equal?(x=5, y=w967) -> (x = y?=w970:bool)
                  n320 = Subtract(x=5, y=w967) -> (x-y=w965:i32)
                  n321 = Number To Decimal String(number=w965) -> (decimal integer string=w966:string)  [unwired: 1 in]
                  n322 = property on="LAMP" class="Bool (strict)"("BoolText.Text"=w966) -> ()  [unwired: 2 in, 2 out]
                }
                n323 = Wait (ms)(milliseconds to wait=u32 5000) -> ()  [unwired: 1 out]
                n324 = call "FLStart.vi"("delay before read (ms)"=w962, "VISA resource name"=w963) -> ("Error Out"=w957:errorcluster, "read buffer"=w958:string)  [unwired: 6 in, 2 out]
                n325 = Match Pattern(string=w958, regular expression=w960) -> (match substring=w961:string)  [unwired: 1 in, 3 out]
                n326 = call <vilib>:"Simple Error Handler.vi"("error source (\" \")"="Lamp" ("error source (\" \")"), "error in (no error)"=w957) -> ()  [unwired: 3 in, 5 out]
                n327 = Equal?(x=w961, y=w960) -> (x = y?=w959:bool)
              }
              frame #1 {
                n328 = case shown="True" w972 {
                  tunnel: ["Flashlamp NOT firing" "Flashlamp activated"] -> w973
                  frame False {
                    n329 = property on="LAMP" class="Bool (strict)"("Value"=FALSE ("LAMP")) -> ()  [unwired: 2 in, 2 out]
                  }
                  frame True {
                    w976 = TRUE ("Visible")
                    n330 = property on="LASER" class="Bool (strict)"("Visible"=w976) -> ()  [unwired: 2 in, 2 out]
                    n331 = property on="Capture" class="Bool"("Visible"=w976) -> ()  [unwired: 2 in, 2 out]
                    n332 = property on="LAMP" class="Bool (strict)"("BoolText.Text"="LAMP ON" ("Boolean Text.Text")) -> ()  [unwired: 2 in, 2 out]
                    n333 = property on="SINGLE SHOT" class="Bool"("Visible"=w976) -> ()  [unwired: 2 in, 2 out]
                  }
                }
              }
            }
          }
        }
      }
      event "LASER": Value Change {
        n334 = event-data() -> ()  [unwired: 1 in, 6 out]
        n335 = case shown="False" "LASER" {
          tunnel: [w993 w1122] -> w983
          tunnel: [w992 w1121] -> w982
          tunnel: w980 -> [w990 w1116]
          tunnel: w979 -> [w989 w1115]
          frame False {
            w987 = "fire" ("regular expression")
            n336 = local read "LAMP"() -> (w991:bool)
            n337 = case shown="True" w991 {
              tunnel: [FALSE ("Visible") TRUE ("Visible")] -> w984
              frame False {
              }
              frame True {
              }
            }
            n338 = property on="Capture" class="Bool"("Visible"=w984) -> ()  [unwired: 2 in, 2 out]
            n339 = property on="SINGLE SHOT" class="Bool"("Visible"=w984) -> ()  [unwired: 2 in, 2 out]
            n340 = call "QSStop.vi"("delay before read (ms)"=w989, "VISA resource name"=w990) -> ("read buffer"=w986:string)  [unwired: 6 in, 3 out]
            n341 = xnode "Match Regular Expression"("input string"=w986, "regular expression"=w987) -> ("whole match"=w988:string)  [unwired: 4 in, 4 out]
            n342 = Equal?(x=w988, y=w987) -> (x = y?=w985:bool)
            n343 = case shown="False" w985 {
              tunnel: [FALSE w997] -> w993
              tunnel: ["" "Q-Switch deactivated"] -> w992
              frame False {
              }
              frame True {
                w997 = FALSE ("Boolean")
                n344 = property on="LASER" class="Bool (strict)"("BoolText.Text"="LASER OFF" ("Boolean Text.Text"), "Value"=w997) -> ()  [unwired: 2 in, 2 out]
                n345 = property on="Laser Operation" class="Bool (strict)"("Blinking"=w997) -> ()  [unwired: 2 in, 2 out]
              }
            }
          }
          frame True {
            w1118 = "fire" ("regular expression")
            n346 = call "CheckStatus.vi"("delay before read (ms)"=w1115, "VISA resource name"=w1116) -> ("read buffer"=w1120:string)  [unwired: 6 in, 3 out]
            n347 = Match Pattern(string=w1120, regular expression=w1118) -> (match substring=w1119:string)  [unwired: 1 in, 3 out]
            n348 = Equal?(x=w1119, y=w1118) -> (x = y?=w1117:bool)
            n349 = case shown="True" w1117 {
              tunnel: [FALSE ("Boolean") w1133] -> w1122
              tunnel: ["The flashlamp is not firing" w1132] -> w1121
              tunnel: w1116 -> [_ w1131]
              tunnel: w1115 -> [_ w1130]
              frame False {
                n350 = property on="LASER" class="Bool (strict)"("Value"=FALSE ("LASER")) -> ()  [unwired: 2 in, 2 out]
              }
              frame True {
                w1128 = "qs" ("regular expression")
                n351 = call "QSStart.vi"("delay before read (ms)"=w1130, "VISA resource name"=w1131) -> ("read buffer"=w1127:string)  [unwired: 6 in, 3 out]
                n352 = Match Pattern(string=w1127, regular expression=w1128) -> (match substring=w1129:string)  [unwired: 1 in, 3 out]
                n353 = Equal?(x=w1129, y=w1128) -> (x = y?=w1126:bool)
                n354 = case shown="True" w1126 {
                  tunnel: [FALSE ("Boolean") w1139] -> w1133
                  tunnel: ["Q-Switch is NOT firing" "Q-Switch activated"] -> w1132
                  frame False {
                    n355 = property on="LASER" class="Bool (strict)"("Value"=FALSE ("LASER")) -> ()  [unwired: 2 in, 2 out]
                  }
                  frame True {
                    w1137 = FALSE ("Visible")
                    w1139 = TRUE ("Boolean")
                    n356 = property on="Capture" class="Bool"("Visible"=w1137) -> ()  [unwired: 2 in, 2 out]
                    n357 = property on="Laser Operation" class="Bool (strict)"("Blinking"=w1139) -> ()  [unwired: 2 in, 2 out]
                    n358 = property on="LASER" class="Bool (strict)"("BoolText.Text"="LASER ON" ("Boolean Text.Text")) -> ()  [unwired: 2 in, 2 out]
                    n359 = property on="SINGLE SHOT" class="Bool"("Visible"=w1137) -> ()  [unwired: 2 in, 2 out]
                  }
                }
              }
            }
          }
        }
        "Laser Operation" <- w983
      }
      event "Repetition\nRate (Hz)": Value Change {
        n360 = event-data() -> ()  [unwired: 1 in, 6 out]
        n361 = call "FLFrequencySet.vi"("Frequency (Hz)"="Repetition\nRate (Hz)", "delay before read (ms)"=w1141, "VISA resource name"=w1142) -> ()  [unwired: 5 in, 4 out]
        n362 = Number To Fractional String(number="Repetition\nRate (Hz)", precision (6)=i16 2 ("width (-)")) -> (F-format string=w1147:string)  [unwired: 2 in]
        n363 = Concatenate Strings("Repetition rate set to: " ("string"), w1147, " Hz" ("string")) -> (w1145:string)
      }
      event "EXIT": Value Change {
        n364 = event-data() -> ()  [unwired: 1 in, 6 out]
        n365 = flat-sequence {
          tunnel: w1150 -> [w1153]
          tunnel: w1149 -> [w1152]
          tunnel: ["EXIT"] -> w1151
          frame #0 {
            n366 = call "QSStop.vi"("delay before read (ms)"=w1152, "VISA resource name"=w1153) -> ("Error Out"=w1154:errorcluster)  [unwired: 6 in, 3 out]
            n367 = call "FLStop.vi"("Error In"=w1154, "delay before read (ms)"=w1152, "VISA resource name"=w1153) -> ()  [unwired: 5 in, 4 out]
          }
          frame #1 {
            n368 = Wait (ms)(milliseconds to wait=u32 1000) -> ()  [unwired: 1 out]
          }
          frame #2 {
            n369 = local write "Camera Status"("Exit camera") -> ()
          }
          frame #3 {
            n370 = Wait (ms)(milliseconds to wait=u32 1000) -> ()  [unwired: 1 out]
          }
          frame #4 {
            n371 = control-ref of="This Application"() -> (w1175:refnum<vi>)
            n372 = call "Personal document path.vi"() -> ("My Documents"=w1158:path)  [unwired: 10 in, 1 out]
            n373 = property class="App"(reference=w1175) -> ("App.Kind"=w1174:T8)  [unwired: 1 in, 2 out]
            n374 = Build Path(base path=w1158, name or relative path="Laser Ablation and Capture - Logs") -> (appended path=w1168:path)
            n375 = case shown="\"Run Time System\"" w1174 {
              frame "Development System", Default {
              }
              frame "Run Time System" {
                n376 = control-ref of="This VI"() -> (w1184:refnum<vi>)
                n377 = invoke class="VI" method="FP.Close"(reference=w1184) -> ()  [unwired: 2 in, 3 out]
                n378 = Quit LabVIEW() -> ()  [unwired: 1 in]
              }
            }
            n379 = call <vilib>:"Check if File or Folder Exists.vi"("path"=w1168) -> ("file or folder exists?"=w1169:bool, "dup path"=w1170:path)  [unwired: 8 in, 1 out]
            n380 = case shown="False" w1169 {
              tunnel: w1170 -> [w1177 w1178]
              tunnel: [w1176 w1178] -> w1173
              frame False {
                n381 = Create Folder(path (use dialog)=w1177) -> (created path=w1176:path)  [unwired: 2 in, 2 out]
              }
              frame True {
              }
            }
            n382 = Get Date/Time In Seconds() -> (seconds since 1Jan1904=w1166:timestamp)
            n383 = Format Date/Time String(time format string (%c)="%d%m%y %I-%M %p ", seconds (now)=w1166) -> (date/time string=w1164:string)  [unwired: 1 in]
            n384 = Concatenate Strings(w1164, "Log File.txt") -> (w1172:string)
            n385 = Build Path(base path=w1173, name or relative path=w1172) -> (appended path=w1171:path)
            n386 = Open/Create/Replace File(file path (use dialog)=w1171, operation (0:open)=T6."replace or create") -> (refnum out=w1162:refnum<file>, cancelled=w1160:bool, error out=w1161:errorcluster)  [unwired: 4 in]
            n387 = case shown="False" w1160 {
              tunnel: w1162 -> [w1183 _]
              tunnel: w1161 -> [w1181 _]
              frame False {
                n388 = local read "Log"() -> (w1182:string)
                n389 = Write to Text File(file (use dialog)=w1183, text=w1182, error in=w1181) -> (refnum out=w1180:refnum<file>, error out=w1179:errorcluster)  [unwired: 2 out]
                n390 = Close File(refnum=w1180, error in=w1179) -> ()  [unwired: 2 out]
              }
              frame True {
              }
            }
          }
          frame #5 {
          }
        }
      }
      event "Log files": Value Change {
        n391 = event-data() -> ()  [unwired: 1 in, 6 out]
        n392 = case shown="True" "Log files" {
          frame False {
          }
          frame True {
            n393 = call "Personal document path.vi"() -> ("My Documents"=w1188:path)  [unwired: 10 in, 1 out]
            n394 = Build Path(base path=w1188, name or relative path="Laser Ablation and Capture - Logs") -> (appended path=w1187:path)
            n395 = Path To String(path=w1187) -> (string=w1193:string)
            n396 = Concatenate Strings("cmd /c explorer.exe " ("string"), w1193) -> (w1191:string)
            n397 = call <vilib>:"System Exec.vi"("run minimized? (F)"=TRUE, "command line"=w1191) -> ()  [unwired: 6 in, 4 out]
          }
        }
      }
      event "Processing time unit", "Processi time (sec)": Value Change {
        n398 = event-data() -> ()  [unwired: 1 in, 6 out]
        n399 = local read "Processing time unit"() -> (w1196:string)
        n400 = Equal?(x=w1196, y="min") -> (x = y?=w1194:bool)
        n401 = case shown="False" w1194 {
          frame False {
            n402 = local read "Processi time (sec)"() -> (w1197:i32)
            n403 = local write "Process time"(w1197) -> ()
          }
          frame True {
            n404 = local read "Processi time (sec)"() -> (w1199:i32)
            n405 = Quotient & Remainder(x=w1199, y=60) -> (floor(x/y)=w1198:i32)  [unwired: 1 out]
            n406 = local write "Process time"(w1198) -> ()
          }
        }
      }
      event "Overlay MSI Image": Value Change {
        n407 = event-data() -> ()  [unwired: 1 in, 6 out]
        n408 = vi-ref "MSI_Image_overlap.vi"() -> (w1201:refnum<vi>)
        n409 = case shown="True" "Overlay MSI Image" {
          tunnel: w1201 -> [_ w1206]
          frame False {
          }
          frame True {
            n410 = invoke class="VI" method="FP.Open"(reference=w1206, "Activate"=TRUE ("Activate?"), "State"=T7."Standard") -> (reference out=w1209:refnum<vi>, error out=w1204:errorcluster)  [unwired: 2 in, 3 out]
            n411 = invoke class="VI" method="Run VI"(reference=w1209, error in=w1204, "Wait until done"=FALSE ("Wait Until Done"), "Auto Dispose Ref"=TRUE ("Auto Dispose Reference")) -> (reference out=w1205:refnum<vi>, error out=w1203:errorcluster)  [unwired: 1 in, 3 out]
            n412 = Close Reference(reference=w1205, error in (no error)=w1203) -> ()  [unwired: 1 out]
          }
        }
      }
      event "SINGLE SHOT": Value Change {
        n413 = event-data() -> ()  [unwired: 1 in, 6 out]
        n414 = case shown="True" "SINGLE SHOT" {
          tunnel: w1215 -> [_ w1219]
          tunnel: w1214 -> [_ w1218]
          tunnel: ["" w1217] -> w1212
          frame False {
          }
          frame True {
            w1223 = "fire" ("regular expression")
            n415 = call "CheckStatus.vi"("delay before read (ms)"=w1218, "VISA resource name"=w1219) -> ("read buffer"=w1221:string)  [unwired: 6 in, 3 out]
            n416 = Match Pattern(string=w1221, regular expression=w1223) -> (match substring=w1222:string)  [unwired: 1 in, 3 out]
            n417 = Equal?(x=w1222, y=w1223) -> (x = y?=w1220:bool)
            n418 = case shown="True" w1220 {
              tunnel: ["The flashlamp is not firing" w1231] -> w1217
              tunnel: w1219 -> [_ w1230]
              tunnel: w1218 -> [_ w1229]
              frame False {
              }
              frame True {
                w1227 = "qs" ("regular expression")
                n419 = call "QSSingleShot.vi"("delay before read (ms)"=w1229, "VISA resource name"=w1230) -> ("read buffer"=w1226:string)  [unwired: 6 in, 3 out]
                n420 = Match Pattern(string=w1226, regular expression=w1227) -> (match substring=w1228:string)  [unwired: 1 in, 3 out]
                n421 = Equal?(x=w1228, y=w1227) -> (x = y?=w1225:bool)
                n422 = case shown="True" w1225 {
                  tunnel: ["Q-Switch is NOT firing" "Q-Switch activated"] -> w1231
                  frame False {
                  }
                  frame True {
                  }
                }
              }
            }
          }
        }
      }
      event "Laser Status": Value Change {
        n423 = event-data() -> ()  [unwired: 1 in, 6 out]
        n424 = case shown="True" "Laser Status" {
          tunnel: w1235 -> [_ w1238]
          tunnel: w1234 -> [_ w1237]
          frame False {
          }
          frame True {
            n425 = call "ICE450UltraMonitor.vi"("delay before read (ms)"=w1237, "VISA resource name"=w1238) -> ()  [unwired: 10 in]
          }
        }
      }
      event "Open \nManual": Value Change {
        n426 = event-data() -> ()  [unwired: 1 in, 6 out]
        n427 = case shown="True" "Open \nManual" {
          tunnel: [_ "Opening Manual" ("StringOut")] -> w1240
          frame False {
          }
          frame True {
            w1249 = FALSE  # wait until completion? (T)
            n428 = control-ref of="This VI"() -> (w1253:refnum<vi>)
            n429 = property class="VI"(reference=w1253) -> ("Path"=w1252:path)  [unwired: 1 in, 2 out]
            n430 = Strip Path(path=w1252) -> (stripped path=w1251:path)  [unwired: 1 out]
            n431 = Build Path(base path=w1251, name or relative path="LAST_Software_Manual.PDF") -> (appended path=w1243:path)
            n432 = Path To String(path=w1243) -> (string=w1246:string)
            n433 = Concatenate Strings("cmd  /c \"", w1246, "\"" ("string")) -> (w1241:string)
            n434 = call <vilib>:"System Exec.vi"("run minimized? (F)"=TRUE, "wait until completion? (T)"=w1249, "error in (no error)"="error in (no error)", "command line"=w1241) -> ("error out"=→"error out":errorcluster)  [unwired: 4 in, 3 out]
          }
        }
      }
      event "Stages status": Value Change {
        w1261 = "Ready"
        n435 = event-data() -> ()  [unwired: 1 in, 6 out]
        n436 = case shown="True" "Stages status" {
          tunnel: w1270 -> [_ w1283]
          tunnel: w1269 -> [_ w1282]
          tunnel: w1268 -> [_ w1281]
          tunnel: [w1274 w1280] -> w1267
          tunnel: [w1274 w1278] -> w1257
          tunnel: [w1274 w1279] -> w1256
          frame False {
            w1274 = ""
          }
          frame True {
            n437 = call <userlib>:"Open TCP-IP.vi"("IP address"=w1283) -> ("error out"=w1277:errorcluster, "Connection ID"=w1284:T9)  [unwired: 8 in, 1 out]
            n438 = call <vilib>:"Simple Error Handler.vi"("error in (no error)"=w1277) -> ("error?"=w1275:bool, "error out"=w1276:errorcluster)  [unwired: 4 in, 3 out]
            n439 = case shown="False" w1275 {
              tunnel: w1284 -> [w1305 _]
              tunnel: w1276 -> [w1304 _]
              tunnel: w1282 -> [w1297 _]
              tunnel: w1281 -> [w1296 _]
              tunnel: [w1295 w1306] -> w1280
              tunnel: [w1292 w1306] -> w1279
              tunnel: [w1288 w1306] -> w1278
              frame False {
                n440 = call "Get Stages Status.vi"("error in (no error)"=w1304, "Group Name (250 c max)"=w1297, "connection ID in"=w1305) -> ("error out"=w1301:errorcluster, "XPS error out"=w1300:errorcluster, "Group Status String"=w1292:string, "connection ID out"=w1303:T9)  [unwired: 4 in, 1 out]
                n441 = call "Get Stages Status.vi"("error in (no error)"=w1301, "XPS error in (no error)"=w1300, "Group Name (250 c max)"=w1296, "connection ID in"=w1303) -> ("error out"=w1298:errorcluster, "XPS error out"=w1294:errorcluster, "Group Status String"=w1288:string, "connection ID out"=w1299:T9)  [unwired: 3 in, 1 out]
                n442 = call <vilib>:"Simple Error Handler.vi"("error source (\" \")"="Stage status" ("error source (\" \")"), "error in (no error)"=w1294) -> ()  [unwired: 3 in, 5 out]
                n443 = Concatenate Strings("Axis 1 " ("string"), w1292) -> (w1291:string)
                n444 = call <userlib>:"Close TCP-IP.vi"("error in (no error)"=w1298, "connection ID in"=w1299) -> ("Error out"=w1293:errorcluster)  [unwired: 9 in]
                n445 = call <vilib>:"Simple Error Handler.vi"("error source (\" \")"="TCP close Stage status" ("error source (\" \")"), "error in (no error)"=w1293) -> ()  [unwired: 3 in, 5 out]
                n446 = Concatenate Strings("Axis 2 " ("string"), w1288) -> (w1289:string)
                n447 = Concatenate Strings(w1291, " - " ("string"), w1289) -> (w1295:string)
              }
              frame True {
                w1306 = ""
              }
            }
          }
        }
        n448 = String Subset(string=w1256, offset (0)=0, length (rest)=5 ("length (rest)")) -> (substring=w1260:string)
        n449 = String Subset(string=w1257, offset (0)=0, length (rest)=5 ("length (rest)")) -> (substring=w1262:string)
        n450 = Equal?(x=w1261, y=w1260) -> (x = y?=w1258:bool)
        n451 = Equal?(x=w1262, y=w1261) -> (x = y?=w1259:bool)
        n452 = And(x=w1259, y=w1258) -> (x .and. y?=w1255:bool)
        n453 = case shown="True" w1255 {
          frame False {
          }
          frame True {
            n454 = property on="Axes Manual Control" class="Bool (strict)"("Visible"=TRUE) -> ()  [unwired: 2 in, 2 out]
            n455 = property on="Home Axes" class="Bool"("Visible"=TRUE) -> ()  [unwired: 2 in, 2 out]
          }
        }
      }
      event "Save configuration": Value Change {
        n456 = event-data() -> ()  [unwired: 1 in, 6 out]
        n457 = case shown="True" "Save configuration" {
          frame False {
          }
          frame True {
            n458 = control-ref of="This VI"() -> (w1329:refnum<vi>)
            n459 = local read "Pixelclock"() -> (w1310:i32)
            n460 = local read "Framerate"() -> (w1309:dbl)
            n461 = local read "Exposure"() -> (w1308:dbl)
            n462 = property class="VI"(reference=w1329) -> ("Path"=w1328:path)  [unwired: 1 in, 2 out]
            n463 = Strip Path(path=w1328) -> (stripped path=w1327:path)  [unwired: 1 out]
            n464 = local read "Height \nstep divider"() -> (w1322:i32)
            n465 = Build Path(base path=w1327, name or relative path="General_Configuration.ini") -> (appended path=w1325:path)
            n466 = local read "Speed (µm/s)"() -> (w1318:i32)
            n467 = local read "Precision (%)"() -> (w1319:dbl)
            n468 = local read "Heigth (px)"() -> (w1321:i32)
            n469 = local read "Width (px)"() -> (w1317:i32)
            n470 = local read "Pixel size"() -> (w1320:dbl)
            n471 = local read "Y offset"() -> (w1316:i32)
            n472 = local read "X travel"() -> (w1314:dbl)
            n473 = local read "X offset"() -> (w1315:i32)
            n474 = local read "Y travel"() -> (w1313:dbl)
            n475 = call <vilib>:"Open Config Data.vi"("create file if necessary (T)"=FALSE, "configuration file path"=w1325) -> ("error out"=w1312:errorcluster, "refnum"=w1323:T5)  [unwired: 7 in, 1 out]
            n476 = call "Configuration writer.vi"("Path"=w1323, "Width (px)"=w1317, "error in (no error)"=w1312, "Precision (%)"=w1319, "Heigth (px)"=w1321, "X offset"=w1316, "X travel"=w1314, "Y offset"=w1315, "Speed (µm/s)"=w1318, "Height  step \ndivider"=w1322, "Y travel"=w1313, "Pixel size"=w1320, "Pixelclock"=w1310, "Framerate"=w1309, "Exposure"=w1308) -> ("error out"=w1311:errorcluster)  [unwired: 4 in]
            n477 = call <vilib>:"Simple Error Handler.vi"("error in (no error)"=w1311) -> ()  [unwired: 4 in, 5 out]
          }
        }
      }
      event "Process Image": Value Change {
        n478 = event-data() -> ()  [unwired: 1 in, 6 out]
        n479 = case shown="True" "Process Image" {
          tunnel: ["" "Processing done"] -> w1331
          frame False {
          }
          frame True {
            (unwired) "untitled" ("Image Name")
            w1364 = 0.2  # Delay after laser on/off
            w1433 = T10 0 items=["Grayscale (U8)", "Grayscale (I16)", "Grayscale (SGL)", "Complex (CSG)", "RGB (U32)", "HSL (U32)", "RGB (U64)", "Grayscale (U16)"] ("Image Type")
            w1436 = i16 6 ("precision (6)")
            w1430 = 1000 ("y")
            n480 = control-ref of="This VI"() -> (w1340:refnum<vi>)
            n481 = control-ref of="This VI"() -> (w1348:refnum<vi>)
            n482 = call "IMAQ Create"("Image Name"="untitled") -> ("New Image"=w1338:T2, "error out"=w1335:errorcluster)  [unwired: 4 in]
            n483 = local read "Source"() -> (w1435:T2)
            n484 = property class="VI"(reference=w1348) -> ("Path"=w1347:path)  [unwired: 1 in, 2 out]
            n485 = Strip Path(path=w1347) -> (stripped path=w1346:path)  [unwired: 1 out]
            n486 = property on="Source" class="ImageControl"() -> ("ROI"=w1336:T11)  [unwired: 2 in, 2 out]
            n487 = call "IMAQ ROIToMask 2"("error in (no error)"=w1335, "ROI Descriptor"=w1336, "Image"=w1338) -> ("error out"=w1334:errorcluster, "Image Out"=w1337:T2)  [unwired: 6 in, 1 out]
            n488 = property class="VI"(reference=w1340, error in=w1334) -> (error out=w1333:errorcluster, "Path"=w1341:path)  [unwired: 1 out]
            n489 = Strip Path(path=w1341) -> (stripped path=w1342:path)  [unwired: 1 out]
            n490 = call "IMAQ Cast Image"("Image Type"=w1433, "Image Src"=w1435) -> ("error out"=w1404:errorcluster, "Image Dst Out"=w1434:T2)  [unwired: 8 in]
            n491 = Unbundle By Name(w1336) -> ("Global Rectangle"=w1383:i32[])
            n492 = Build Path(base path=w1342, name or relative path="Last_ROI.TIFF") -> (appended path=w1344:path)
            n493 = call-poly "IMAQ Write File 2"("error in (no error)"=w1333, "File Path"=w1344, "Image"=w1337) -> ()  [unwired: 7 in, 2 out]
            n494 = Build Path(base path=w1346, name or relative path="Last_ROI.TIFF") -> ()  [unwired: 1 out]
            n495 = call "IMAQ ROIToMask 2"("error in (no error)"=w1404, "ROI Descriptor"=w1336, "Image"=w1434) -> ("error out"=w1405:errorcluster, "Image Out"=w1437:T2)  [unwired: 6 in, 1 out]
            n496 = call "IMAQ ImageToArray"("error in (no error)"=w1405, "Image"=w1437) -> ("error out"=w1403:errorcluster, "Image Pixels (U8)"=w1380:u8[][])  [unwired: 2 in, 3 out]
            n497 = Array To Cluster(array=w1383) -> (cluster=w1406:T12)
            n498 = Unbundle(w1406) -> ("Global Rectangle[0]"=w1359:i32, "Global Rectangle[1]"=w1360:i32)
            n499 = call <vilib>:"Simple Error Handler.vi"("error in (no error)"=w1403) -> ()  [unwired: 4 in, 5 out]
            n500 = local read "X offset"() -> (w1398:i32)
            n501 = local read "Y offset"() -> (w1397:i32)
            n502 = Subtract(x=w1360, y=w1397) -> (x-y=w1387:i32)
            n503 = Subtract(x=w1359, y=w1398) -> (x-y=w1388:i32)
            n504 = local read "Width (px)"() -> (w1389:i32)
            n505 = call "ROI corrector.vi"("ROI"=w1380, "Spot diameter"=w1389) -> ("Corrected ROI"=w1386:u8[][])  [unwired: 9 in]
            n506 = Add Array Elements(numeric array=w1386) -> (sum=w1385:u8)
            n507 = Less Or Equal To 0?(x=w1385) -> (x <= 0?=w1384:bool)
            n508 = case shown="False" w1384 {
              tunnel: [w1448 u8[][] [[1]] ("Image Pixels (U8)")] -> w1423
              tunnel: w1386 -> [w1448 _]
              frame False {
              }
              frame True {
                n509 = One Button Dialog(message="ATTENTION: you did not select\nany region of interest") -> ()  [unwired: 1 in, 1 out]
              }
            }
            n510 = local read "Heigth (px)"() -> (w1375:i32)
            n511 = Divide(x=w1389, y=2) -> (x/y=w1393:dbl)
            n512 = Initialize Array(1 ("element"), w1389, w1389) -> (w1394:i32[][])
            n513 = Round To Nearest(number=w1393) -> (nearest integer value=w1382:dbl)
            n514 = call "Circle Spot Calculator.vi"("Center Y"=w1382, "Radius"=w1382, "Center X"=w1382, "initialized array"=w1394) -> ("Array"=w1391:i32[][])  [unwired: 6 in]
            n515 = Array Size(array=w1380) -> (size(s)=w1379:i32[])
            n516 = local read "Pixel size"() -> (w1399:dbl)
            n517 = Add Array Elements(numeric array=w1391) -> (sum=w1390:i32)
            n518 = Array To Cluster(array=w1379) -> (cluster=w1381:cluster{"[0]":i32, "[1]":i32})
            n519 = Multiply(x=w1388, y=w1399) -> (x*y=w1400:dbl)
            n520 = Unbundle(w1381) -> ("[0]"=w1378:i32, "[1]"=w1377:i32)
            "Rect width\n(px)" <- w1377
            "Rect height\n(px)" <- w1378
            n521 = Multiply(x=w1399, y=w1387) -> (x*y=w1401:dbl)
            n522 = Multiply(x=w1399, y=w1399) -> (x*y=w1426:dbl)
            n523 = To Double Precision Float(number=w1423) -> (double precision float=w1424:dbl[][])
            n524 = local read "Height \nstep divider"() -> (w1374:i32)
            n525 = Divide(x=w1401, y=w1430) -> (x/y=w1432:dbl)
            n526 = Divide(x=w1400, y=w1430) -> (x/y=w1431:dbl)
            n527 = Add Array Elements(numeric array=w1424) -> (sum=w1428:dbl)
            n528 = local read "Axis 2 inverted?"() -> (w1368:bool)
            n529 = local read "Axis 1 inverted?"() -> (w1369:bool)
            n530 = Number To Fractional String(number=w1432, precision (6)=w1436) -> (F-format string=w1421:string)  [unwired: 2 in]
            n531 = Number To Fractional String(number=w1431, precision (6)=w1436) -> (F-format string=w1422:string)  [unwired: 2 in]
            n532 = Divide(x=w1428, y=u8 255) -> (x/y=w1425:dbl)
            n533 = Multiply(x=w1425, y=w1426) -> (x*y=w1420:dbl)
            n534 = Multiply(x=w1378, y=w1399) -> (x*y=w1416:dbl)
            n535 = Multiply(x=w1377, y=w1399) -> (x*y=w1417:dbl)
            n536 = Fract/Exp String To Number(string=w1421) -> (number=w1373:dbl)  [unwired: 3 in, 1 out]
            n537 = Fract/Exp String To Number(string=w1422) -> (number=w1372:dbl)  [unwired: 3 in, 1 out]
            n538 = Divide "Height of a line"(x=w1375, y=w1374) -> (x/y=w1408:dbl)
            n539 = Multiply(x=w1399, y=w1408) -> (x*y=w1409:dbl)
            n540 = Round To Nearest(number=w1416) -> (nearest integer value=→"Rect height\n(µm/px)":dbl)
            n541 = Round To Nearest(number=w1417) -> (nearest integer value=→"Rect. width \n(µm/px))":dbl)
            n542 = case shown="True" w1368 {
              tunnel: w1372 -> [w1442 w1444]
              tunnel: [w1442 w1443] -> w1370
              frame False {
              }
              frame True {
                n543 = Negate(x=w1444) -> (-x=w1443:dbl)
              }
            }
            "Axis 2 Offset" <- w1370
            n544 = case shown="True" w1369 {
              tunnel: w1373 -> [w1445 w1447]
              tunnel: [w1445 w1446] -> w1371
              frame False {
              }
              frame True {
                n545 = Negate(x=w1447) -> (-x=w1446:dbl)
              }
            }
            "Axis 1 Offset" <- w1371
            n546 = Divide(x=w1420, y=1000000.0) -> (x/y=→"ROI Area \n(mm2)":dbl)
            n547 = call "ROI parser.vi"("Circle spot"=w1390, "Circle?"="Circle?", "ROI (8 bit image)"=w1423, "Ablation spot width"=w1389, "Sampling\nPrecision"="Precision (%)", "Ablation spot heigth"=w1375, "Height  step \ndivider"=w1374) -> ("Parsed array"=w1441:bool[][])  [unwired: 4 in]
            n548 = call "Array processor.vi"("Source array"=w1441, "Pixel size"=w1399) -> ("Lenght array"=w1402:dbl[][], "T/F product array"=w1412:bool[][])  [unwired: 8 in]
            n549 = Index Array(array=w1412, index (col)=0 ("disabled index (col)")) -> (element=w1439:bool[])  [unwired: 1 in]
            n550 = Array Size(array=w1439) -> (size(s)=w1438:i32)
            n551 = for {
              N: w1438 -> [_]
              tunnel: w1412 -> [w1453] mode=indexing
              tunnel: [w1451] -> w1367 mode=indexing
              # "This loop add a F for each Y moviment"
              n552 = Build Array (concatenate)(w1453, FALSE) -> (w1451:bool[])
            }
            "Laser on/off array" <- w1367
            n553 = Round To Nearest(number=w1409) -> (nearest integer value=w1407:dbl)
            n554 = local read "Speed (µm/s)"() -> (w1413:i32)
            n555 = Boolean To (0,1)(Boolean=w1367) -> (0, 1=w1366:i16[][])
            n556 = Add Array Elements(numeric array=w1366) -> (sum=w1365:i16)
            n557 = Multiply(x=w1364, y=w1365) -> (x*y=w1362:dbl)
            n558 = local read "Axis 1"() -> (w1415:string)
            n559 = local read "Axis 2"() -> (w1414:string)
            n560 = call "Commands array generator.vi"("Axis 1"=w1415, "Axis 1 inverted?"=w1369, "Axis in"=w1414, "Axis 2 inverted?"=w1368, "Axes speed \n(µm/s)"=w1413, "Y Step size in µm"=w1407, "T/F product array"=w1412, "Space defined array"=w1402) -> ("Command Array"=w1358:string[][], "Time Array"=w1363:dbl[][])  [unwired: 2 in]
            "Commands array" <- w1358
            n561 = Add Array Elements(numeric array=w1363) -> (sum=w1361:dbl)
            n562 = Array Size(array=w1358) -> (size(s)=w1357:i32[])
            n563 = Add(x=w1362, y=w1361) -> (x+y=w1350:dbl)
            n564 = Array To Cluster(array=w1357) -> (cluster=w1356:cluster{"[0]":i32, "[1]":i32})
            n565 = Unbundle(w1356) -> ("[0]"=w1355:i32, "[1]"=w1354:i32)
            n566 = Multiply(x=w1355, y=w1354) -> (x*y=w1352:i32)
            n567 = Multiply(x="Captur time\nConstant", y=w1352) -> (x*y=w1351:dbl)
            n568 = Add(x=w1350, y=w1351) -> (x+y=w1349:dbl)
            "Processi time (sec)" <- w1349
            n569 = local write "Process time"(w1349) -> ()
          }
        }
      }
      event "Call Last ROI": Value Change {
        n570 = event-data() -> ()  [unwired: 1 in, 6 out]
        n571 = control-ref of="This VI"() -> (w1454:refnum<vi>)
        n572 = property class="VI"(reference=w1454) -> ("Path"=w1457:path)  [unwired: 1 in, 2 out]
        n573 = Strip Path(path=w1457) -> (stripped path=w1456:path)  [unwired: 1 out]
        n574 = Build Path(base path=w1456, name or relative path="Last_ROI.TIFF") -> (appended path=w1460:path)
        n575 = call <vilib>:"Check if File or Folder Exists.vi"("path"=w1460) -> ("file or folder exists?"=w1459:bool)  [unwired: 8 in, 2 out]
        n576 = And(x=w1459, y="Call Last ROI") -> (x .and. y?=w1461:bool)
        n577 = case shown="True" w1461 {
          tunnel: w1460 -> [_ w1469]
          frame False {
          }
          frame True {
            n578 = call "IMAQ Create"("Image Name"="untitled") -> ("New Image"=w1471:T2)  [unwired: 4 in, 1 out]
            n579 = call "IMAQ ReadFile"("File Path"=w1469, "Image"=w1471) -> ("Image Out"=w1470:T2)  [unwired: 5 in, 4 out]
            n580 = call "IMAQ MaskToROI"("Image"=w1470) -> ("ROI Descriptor"=w1462:T13)  [unwired: 6 in, 2 out]
            n581 = Unbundle By Name(w1462) -> ("Contours"=w1467:T14)  [unwired: 1 out]
            n582 = Index Array(array=w1467) -> (element=w1468:T15)  [unwired: 1 in]
            n583 = Bundle By Name(cluster=w1468, "Type"=u32 6) -> (w1466:T15)
            n584 = Replace Array Subset(array=w1467, new element=w1466) -> (w1465:T14)  [unwired: 1 in]
            n585 = Bundle By Name(cluster=w1462, "Contours"=w1465) -> (w1463:T13)
            n586 = property on="Source" class="ImageControl"("ROI"=w1463) -> ()  [unwired: 2 in, 2 out]
          }
        }
      }
      event "Save current ROI": Value Change {
        n587 = event-data() -> ()  [unwired: 1 in, 6 out]
        n588 = property on="Source" class="ImageControl"() -> ("ROI"=w1478:T11)  [unwired: 2 in, 2 out]
        n589 = Unbundle By Name(w1478) -> ("Contours"=w1473:T16)
        n590 = Index Array(array=w1473) -> (element=w1474:T17)  [unwired: 1 in]
        n591 = Unbundle By Name(w1474) -> ("ROI Type"=w1475:u32)
        n592 = Not Equal To 0?(x=w1475) -> (x != 0?=w1476:bool)
        n593 = And(x="Save current ROI", y=w1476) -> (x .and. y?=w1479:bool)
        n594 = case shown="True" w1479 {
          tunnel: w1478 -> [_ w1490]
          frame False {
          }
          frame True {
            n595 = control-ref of="This VI"() -> (w1494:refnum<vi>)
            n596 = property class="VI"(reference=w1494) -> ("Path"=w1495:path)  [unwired: 1 in, 2 out]
            n597 = call "IMAQ Create"("Image Name"="untitled") -> ("New Image"=w1491:T2)  [unwired: 4 in, 1 out]
            n598 = call "IMAQ ROIToMask 2"("ROI Descriptor"=w1490, "Image"=w1491) -> ("Image Out"=w1493:T2)  [unwired: 7 in, 2 out]
            n599 = Strip Path(path=w1495) -> (stripped path=w1496:path)  [unwired: 1 out]
            n600 = Build Path(base path=w1496, name or relative path="Saved ROI") -> (appended path=w1489:path)
            n601 = call <vilib>:"Check if File or Folder Exists.vi"("path"=w1489) -> ("file or folder exists?"=w1488:bool, "dup path"=w1487:path)  [unwired: 8 in, 1 out]
            n602 = case shown="True" w1488 {
              tunnel: w1487 -> [w1499 w1500]
              tunnel: [w1498 w1500] -> w1486
              frame False {
                n603 = Create Folder(path (use dialog)=w1499) -> (created path=w1498:path)  [unwired: 2 in, 2 out]
              }
              frame True {
              }
            }
            n604 = Get Date/Time In Seconds() -> (seconds since 1Jan1904=w1483:timestamp)
            n605 = Format Date/Time String(time format string (%c)="%d%m%y %I-%M %p ", seconds (now)=w1483) -> (date/time string=w1482:string)  [unwired: 1 in]
            n606 = Concatenate Strings(w1482, " - saved ROI.tiff" ("string")) -> (w1480:string)
            n607 = Build Path(base path=w1486, name or relative path=w1480) -> (appended path=w1485:path)
            n608 = call-poly "IMAQ Write File 2"("File Path"=w1485, "Image"=w1493) -> ()  [unwired: 8 in, 2 out]
          }
        }
      }
      event "Load ROI": Value Change {
        n609 = event-data() -> ()  [unwired: 1 in, 6 out]
        n610 = case shown="True" "Load ROI" {
          frame False {
          }
          frame True {
            n611 = call "File Dialog"("prompt"="Select an ROI file..." ("pattern label"), "pattern (all files)"="*.jpg;*.bmp;*.jpeg;*.tif;*.tiff;*.png", "pattern label"="ROI files") -> ("selected path"=w1502:path, "cancelled"=w1503:bool)  [unwired: 9 in, 2 out]
            n612 = case shown="False" w1503 {
              tunnel: w1502 -> [w1514 _]
              frame False {
                n613 = call "IMAQ Create"("Image Name"="untitled") -> ("New Image"=w1516:T2)  [unwired: 4 in, 1 out]
                n614 = call "IMAQ ReadFile"("File Path"=w1514, "Image"=w1516) -> ("Image Out"=w1515:T2)  [unwired: 5 in, 4 out]
                n615 = call "IMAQ MaskToROI"("Image"=w1515) -> ("ROI Descriptor"=w1507:T13)  [unwired: 6 in, 2 out]
                n616 = Unbundle By Name(w1507) -> ("Contours"=w1512:T14)  [unwired: 1 out]
                n617 = Index Array(array=w1512) -> (element=w1513:T15)  [unwired: 1 in]
                n618 = Bundle By Name(cluster=w1513, "Type"=u32 6) -> (w1511:T15)
                n619 = Replace Array Subset(array=w1512, new element=w1511) -> (w1510:T14)  [unwired: 1 in]
                n620 = Bundle By Name(cluster=w1507, "Contours"=w1510) -> (w1508:T13)
                n621 = property on="Source" class="ImageControl"("ROI"=w1508) -> ()  [unwired: 2 in, 2 out]
              }
              frame True {
              }
            }
          }
        }
      }
      event "Axes Manual Control": Value Change {
        n622 = event-data() -> ()  [unwired: 1 in, 6 out]
        n623 = case shown="True" "Axes Manual Control" {
          tunnel: w1520 -> [_ w1532]
          tunnel: w1519 -> [_ w1531]
          tunnel: w1518 -> [_ w1530]
          frame False {
          }
          frame True {
            n624 = flat-sequence {
              tunnel: w1532 -> [w1542]
              tunnel: w1531 -> [w1541]
              tunnel: w1530 -> [w1540]
              tunnel: [w1542] -> w1529
              tunnel: [w1541] -> w1528
              tunnel: [w1540] -> w1527
              tunnel: [w1539] -> w1526
              tunnel: [w1538] -> w1525
              tunnel: [w1537] -> w1524
              tunnel: [w1536] -> w1523
              tunnel: w1529 -> [w1585]
              tunnel: w1528 -> [w1584]
              tunnel: w1527 -> [w1583]
              tunnel: w1526 -> [w1578]
              tunnel: w1525 -> [w1577]
              tunnel: w1524 -> [w1568]
              tunnel: w1523 -> [w1567]
              frame #0 {
                n625 = call <userlib>:"Open TCP-IP.vi"("IP address"=w1542) -> ("error out"=w1534:errorcluster, "Connection ID"=w1543:T9)  [unwired: 8 in, 1 out]
                n626 = call <vilib>:"Simple Error Handler.vi"("error in (no error)"=w1534) -> ("error?"=w1533:bool, "error out"=w1535:errorcluster)  [unwired: 4 in, 3 out]
                n627 = case shown="True" w1533 {
                  tunnel: w1543 -> [w1558 _]
                  tunnel: w1535 -> [w1557 _]
                  tunnel: w1541 -> [w1554 _]
                  tunnel: w1540 -> [w1553 _]
                  tunnel: [w1552 w1562] -> w1539
                  tunnel: [w1551 w1562] -> w1538
                  tunnel: [w1547 w1561] -> w1537
                  tunnel: [w1546 w1561] -> w1536
                  frame False {
                    n628 = call "Get Stages Status.vi"("error in (no error)"=w1557, "Group Name (250 c max)"=w1554, "connection ID in"=w1558) -> ("error out"=w1556:errorcluster, "XPS error out"=w1555:errorcluster, "Group Status String"=w1551:string, "connection ID out"=w1550:T9, "Status"=w1546:i32)  [unwired: 4 in]
                    n629 = call "Get Stages Status.vi"("error in (no error)"=w1556, "XPS error in (no error)"=w1555, "Group Name (250 c max)"=w1553, "connection ID in"=w1550) -> ("error out"=w1560:errorcluster, "XPS error out"=w1549:errorcluster, "Group Status String"=w1552:string, "connection ID out"=w1559:T9, "Status"=w1547:i32)  [unwired: 3 in]
                    n630 = call <vilib>:"Simple Error Handler.vi"("error source (\" \")"="Axis manual control check" ("error source (\" \")"), "error in (no error)"=w1549) -> ()  [unwired: 3 in, 5 out]
                    n631 = call <userlib>:"Close TCP-IP.vi"("error in (no error)"=w1560, "connection ID in"=w1559) -> ("Error out"=w1548:errorcluster)  [unwired: 9 in]
                    n632 = call <vilib>:"Simple Error Handler.vi"("error source (\" \")"="TCP close Axis manual control check" ("error source (\" \")"), "error in (no error)"=w1548) -> ()  [unwired: 3 in, 5 out]
                  }
                  frame True {
                    w1561 = 0
                    w1562 = ""
                  }
                }
              }
              frame #1 {
                w1571 = 47 ("y")
                w1572 = "Ready"
                n633 = String Subset(string=w1577, offset (0)=0, length (rest)=5 ("length (rest)")) -> (substring=w1574:string)
                n634 = String Subset(string=w1578, offset (0)=0, length (rest)=5 ("length (rest)")) -> (substring=w1573:string)
                n635 = Equal?(x=w1574, y=w1572) -> (x = y?=w1575:bool)
                n636 = Equal?(x=w1572, y=w1573) -> (x = y?=w1576:bool)
                n637 = Equal?(x=w1571, y=w1567) -> (x = y?=w1569:bool)
                n638 = Equal?(x=w1568, y=w1571) -> (x = y?=w1570:bool)
                n639 = And(x=w1570, y=w1569) -> (x .and. y?=w1564:bool)
                n640 = And(x=w1575, y=w1576) -> (x .and. y?=w1565:bool)
                n641 = Not(x=w1564) -> (.not. x?=w1563:bool)
                n642 = And(x=w1565, y=w1563) -> (x .and. y?=w1566:bool)
                n643 = case shown="True" w1566 {
                  tunnel: w1585 -> [_ w1593]
                  tunnel: w1584 -> [_ w1592]
                  tunnel: w1583 -> [_ w1591]
                  tunnel: w1563 -> [w1586 _]
                  frame False {
                    n644 = case shown="False" w1586 {
                      frame False {
                        n645 = One Button Dialog(message="One or more axis already in jogging position") -> ()  [unwired: 1 in, 1 out]
                      }
                      frame True {
                        n646 = One Button Dialog(message="Axes are not ready") -> ()  [unwired: 1 in, 1 out]
                      }
                    }
                  }
                  frame True {
                    n647 = local read "Axis 2 inverted?"() -> (w1590:bool)
                    n648 = local read "Axis 1 inverted?"() -> (w1589:bool)
                    n649 = call "XPS Controller.vi"("Axis 2"=w1591, "Axis 1"=w1592, "Controller Address"=w1593, "Axis 2 \ninverted?"=w1590, "Axis 1 \ninverted?"=w1589) -> ()  [unwired: 6 in]
                  }
                }
              }
            }
          }
        }
      }
      event "Home Axes": Value Change {
        n650 = event-data() -> ()  [unwired: 1 in, 6 out]
        n651 = flat-sequence {
          tunnel: w1600 -> [w1606]
          tunnel: w1601 -> [w1607]
          tunnel: w1602 -> [w1608]
          tunnel: "Home Axes" -> [w1609]
          tunnel: [w1609] -> w1598
          tunnel: [w1608] -> w1597
          tunnel: [w1607] -> w1596
          tunnel: [w1606] -> w1595
          tunnel: [w1605] -> w1594
          tunnel: [w1613] -> w1599
          tunnel: w1598 -> [w1611]
          tunnel: w1597 -> [w1616]
          tunnel: w1596 -> [w1614]
          tunnel: w1595 -> [w1615]
          tunnel: w1594 -> [w1612]
          tunnel: [w1695] -> w1603
          tunnel: w1599 -> [w1694]
          frame #0 {
            n652 = call "Display Message to User"() -> ("OK"=w1605:bool)  [unwired: 10 in, 1 out]
          }
          frame #1 {
            n653 = And(x=w1611, y=w1612) -> (x .and. y?=w1610:bool)
            n654 = case shown="True" w1610 {
              tunnel: w1616 -> [_ w1632]
              tunnel: w1614 -> [_ w1633]
              tunnel: w1615 -> [_ w1630]
              tunnel: w1614 -> [_ w1631]
              tunnel: [FALSE w1623] -> w1613
              frame False {
              }
              frame True {
                w1629 = 47 ("y")
                w1645 = "Ready"
                n655 = call <userlib>:"Open TCP-IP.vi"("IP address"=w1632) -> ("error out"=w1618:errorcluster, "Connection ID"=w1636:T9)  [unwired: 8 in, 1 out]
                n656 = call <vilib>:"Simple Error Handler.vi"("error in (no error)"=w1618) -> ("error?"=w1620:bool, "error out"=w1619:errorcluster)  [unwired: 4 in, 3 out]
                n657 = case shown="False" w1620 {
                  tunnel: w1619 -> [w1659 _]
                  tunnel: w1636 -> [w1658 _]
                  tunnel: [w1655 w1664] -> w1635
                  tunnel: [w1654 w1664] -> w1634
                  tunnel: w1633 -> [w1653 _]
                  tunnel: w1630 -> [w1652 _]
                  tunnel: [w1649 w1663] -> w1628
                  tunnel: [w1648 w1663] -> w1627
                  frame False {
                    n658 = call "Get Stages Status.vi"("error in (no error)"=w1659, "Group Name (250 c max)"=w1653, "connection ID in"=w1658) -> ("error out"=w1660:errorcluster, "XPS error out"=w1661:errorcluster, "Group Status String"=w1655:string, "connection ID out"=w1662:T9, "Status"=w1648:i32)  [unwired: 4 in]
                    n659 = call "Get Stages Status.vi"("error in (no error)"=w1660, "XPS error in (no error)"=w1661, "Group Name (250 c max)"=w1652, "connection ID in"=w1662) -> ("error out"=w1656:errorcluster, "XPS error out"=w1651:errorcluster, "Group Status String"=w1654:string, "connection ID out"=w1657:T9, "Status"=w1649:i32)  [unwired: 3 in]
                    n660 = call <vilib>:"Simple Error Handler.vi"("error source (\" \")"="home axis check" ("error source (\" \")"), "error in (no error)"=w1651) -> ()  [unwired: 3 in, 5 out]
                    n661 = call <userlib>:"Close TCP-IP.vi"("error in (no error)"=w1656, "connection ID in"=w1657) -> ("Error out"=w1650:errorcluster)  [unwired: 9 in]
                    n662 = call <vilib>:"Simple Error Handler.vi"("error source (\" \")"="TCP close home axis check" ("error source (\" \")"), "error in (no error)"=w1650) -> ()  [unwired: 3 in, 5 out]
                  }
                  frame True {
                    w1663 = 0
                    w1664 = ""
                  }
                }
                n663 = Equal?(x=w1629, y=w1627) -> (x = y?=w1626:bool)
                n664 = Equal?(x=w1628, y=w1629) -> (x = y?=w1625:bool)
                n665 = String Subset(string=w1635, offset (0)=0, length (rest)=5 ("length (rest)")) -> (substring=w1643:string)
                n666 = String Subset(string=w1634, offset (0)=0, length (rest)=5 ("length (rest)")) -> (substring=w1644:string)
                n667 = Equal?(x=w1643, y=w1645) -> (x = y?=w1642:bool)
                n668 = Equal?(x=w1645, y=w1644) -> (x = y?=w1641:bool)
                n669 = And(x=w1625, y=w1626) -> (x .and. y?=w1621:bool)
                n670 = Not(x=w1621) -> (.not. x?=w1622:bool)
                n671 = And(x=w1642, y=w1641) -> (x .and. y?=w1624:bool)
                n672 = And(x=w1624, y=w1622) -> (x .and. y?=w1623:bool)
                n673 = case shown="True" w1623 {
                  tunnel: w1632 -> [_ w1674]
                  tunnel: w1631 -> [_ w1673]
                  tunnel: w1630 -> [_ w1672]
                  tunnel: w1621 -> [w1665 _]
                  frame False {
                    n674 = case shown="True" w1665 {
                      frame False {
                        n675 = One Button Dialog(message="Axes are not ready") -> ()  [unwired: 1 in, 1 out]
                      }
                      frame True {
                        n676 = One Button Dialog(message="One or more axis are in jogging mode") -> ()  [unwired: 1 in, 1 out]
                      }
                    }
                  }
                  frame True {
                    n677 = call <userlib>:"Open TCP-IP.vi"("IP address"=w1674) -> ("error out"=w1690:errorcluster, "Connection ID"=w1691:T9)  [unwired: 8 in, 1 out]
                    n678 = call <userlib>:"Group Kill.vi"("error in (no error)"=w1690, "Group Name (250 c max)"=w1673, "connection ID in"=w1691) -> ("error out"=w1688:errorcluster, "XPS error out"=w1689:errorcluster, "connection ID out"=w1685:T9)  [unwired: 6 in]
                    n679 = call <userlib>:"Group Initialize.vi"("error in (no error)"=w1688, "XPS error in (no error)"=w1689, "Group Name (250 c max)"=w1673, "connection ID in"=w1685) -> ("error out"=w1686:errorcluster, "XPS error out"=w1687:errorcluster, "connection ID out"=w1684:T9)  [unwired: 5 in]
                    n680 = call <userlib>:"Group Home Search.vi"("error in (no error)"=w1686, "XPS error in (no error)"=w1687, "Group Name (250 c max)"=w1673, "connection ID in"=w1684) -> ("error out"=w1675:errorcluster, "XPS error out"=w1676:errorcluster, "connection ID out"=w1683:T9)  [unwired: 5 in]
                    n681 = call <userlib>:"Group Kill.vi"("error in (no error)"=w1675, "XPS error in (no error)"=w1676, "Group Name (250 c max)"=w1672, "connection ID in"=w1683) -> ("error out"=w1677:errorcluster, "XPS error out"=w1678:errorcluster, "connection ID out"=w1682:T9)  [unwired: 5 in]
                    n682 = call <userlib>:"Group Initialize.vi"("error in (no error)"=w1677, "XPS error in (no error)"=w1678, "Group Name (250 c max)"=w1672, "connection ID in"=w1682) -> ("error out"=w1679:errorcluster, "XPS error out"=w1680:errorcluster, "connection ID out"=w1681:T9)  [unwired: 5 in]
                    n683 = call <userlib>:"Group Home Search.vi"("error in (no error)"=w1679, "XPS error in (no error)"=w1680, "Group Name (250 c max)"=w1672, "connection ID in"=w1681) -> ("error out"=w1692:errorcluster, "XPS error out"=w1671:errorcluster, "connection ID out"=w1693:T9)  [unwired: 5 in]
                    n684 = call <vilib>:"Simple Error Handler.vi"("error source (\" \")"="home axis " ("error source (\" \")"), "error in (no error)"=w1671) -> ()  [unwired: 3 in, 5 out]
                    n685 = call <userlib>:"Close TCP-IP.vi"("error in (no error)"=w1692, "connection ID in"=w1693) -> ("Error out"=w1670:errorcluster)  [unwired: 9 in]
                    n686 = call <vilib>:"Simple Error Handler.vi"("error source (\" \")"="TCP close home axis " ("error source (\" \")"), "error in (no error)"=w1670) -> ()  [unwired: 3 in, 5 out]
                  }
                }
              }
            }
          }
          frame #2 {
            n687 = case shown="True" w1694 {
              tunnel: ["" ("StringOut") "Axes have been moved to home position" ("StringOut")] -> w1695
              frame False {
              }
              frame True {
              }
            }
          }
        }
      }
      event "Transparency": Value Change {
        n688 = event-data() -> ()  [unwired: 1 in, 6 out]
        n689 = control-ref of="This VI"() -> (w1699:refnum<vi>)
        n690 = property class="VI"(reference=w1699, "FP:Transparency"="Transparency") -> ()  [unwired: 1 in, 2 out]
      }
      event "Capture": Value Change {
        w1700 = 47 ("y")
        w1726 = "Ready"
        n691 = event-data() -> ()  [unwired: 1 in, 6 out]
        n692 = call <userlib>:"Open TCP-IP.vi"("IP address"=w1714) -> ("error out"=w1703:errorcluster, "Connection ID"=w1717:T9)  [unwired: 8 in, 1 out]
        n693 = call <vilib>:"Simple Error Handler.vi"("error in (no error)"=w1703) -> ("error?"=w1701:bool, "error out"=w1702:errorcluster)  [unwired: 4 in, 3 out]
        n694 = case shown="False" w1701 {
          tunnel: w1702 -> [w1740 _]
          tunnel: w1717 -> [w1739 _]
          tunnel: [w1736 w1744] -> w1716
          tunnel: [w1735 w1744] -> w1715
          tunnel: w1713 -> [w1734 _]
          tunnel: w1712 -> [w1733 _]
          tunnel: [w1731 w1745] -> w1711
          tunnel: [w1730 w1745] -> w1710
          frame False {
            n695 = call "Get Stages Status.vi"("error in (no error)"=w1740, "Group Name (250 c max)"=w1734, "connection ID in"=w1739) -> ("error out"=w1741:errorcluster, "XPS error out"=w1742:errorcluster, "Group Status String"=w1736:string, "connection ID out"=w1743:T9, "Status"=w1730:i32)  [unwired: 4 in]
            n696 = call "Get Stages Status.vi"("error in (no error)"=w1741, "XPS error in (no error)"=w1742, "Group Name (250 c max)"=w1733, "connection ID in"=w1743) -> ("error out"=w1737:errorcluster, "XPS error out"=w1732:errorcluster, "Group Status String"=w1735:string, "connection ID out"=w1738:T9, "Status"=w1731:i32)  [unwired: 3 in]
            n697 = call <vilib>:"Simple Error Handler.vi"("error source (\" \")"="Capture check" ("error source (\" \")"), "error in (no error)"=w1732) -> ()  [unwired: 3 in, 5 out]
            n698 = call <userlib>:"Close TCP-IP.vi"("error in (no error)"=w1737, "connection ID in"=w1738) -> ("Error out"=w1728:errorcluster)  [unwired: 9 in]
            n699 = call <vilib>:"Simple Error Handler.vi"("error in (no error)"=w1728) -> ()  [unwired: 4 in, 5 out]
          }
          frame True {
            w1745 = 0
            w1744 = ""
          }
        }
        n700 = Equal?(x=w1711, y=w1700) -> (x = y?=w1709:bool)
        n701 = Equal?(x=w1700, y=w1710) -> (x = y?=w1708:bool)
        n702 = String Subset(string=w1716, offset (0)=0, length (rest)=5 ("length (rest)")) -> (substring=w1724:string)
        n703 = String Subset(string=w1715, offset (0)=0, length (rest)=5 ("length (rest)")) -> (substring=w1725:string)
        n704 = Equal?(x=w1724, y=w1726) -> (x = y?=w1723:bool)
        n705 = Equal?(x=w1726, y=w1725) -> (x = y?=w1722:bool)
        n706 = And(x=w1709, y=w1708) -> (x .and. y?=w1705:bool)
        n707 = Not(x=w1705) -> (.not. x?=w1704:bool)
        n708 = And(x=w1723, y=w1722) -> (x .and. y?=w1707:bool)
        n709 = And(x=w1707, y=w1704) -> (x .and. y?=w1706:bool)
        n710 = case shown="True" w1706 {
          tunnel: ["" w1771] -> w1727
          tunnel: w1714 -> [_ w1770]
          tunnel: w1712 -> [_ w1769]
          tunnel: w1713 -> [_ w1768]
          tunnel: w1705 -> [w1746 _]
          frame False {
            n711 = case shown="True" w1746 {
              frame False {
                n712 = One Button Dialog(message="Axes are not ready") -> ()  [unwired: 1 in, 1 out]
              }
              frame True {
                n713 = One Button Dialog(message="One or more axis are in jogging mode") -> ()  [unwired: 1 in, 1 out]
              }
            }
          }
          frame True {
            n714 = flat-sequence {
              tunnel: [w1801] -> w1782
              tunnel: [w1787] -> w1781
              tunnel: [w1786] -> w1780
              tunnel: [w1800] -> w1779
              tunnel: [w1799] -> w1778
              tunnel: [w1798] -> w1777
              tunnel: [w1785] -> w1776
              tunnel: w1768 -> [w1796]
              tunnel: w1769 -> [w1797]
              tunnel: w1770 -> [w1785]
              tunnel: [w1784] -> w1757
              tunnel: [w1783] -> w1753
              tunnel: w1782 -> [w1821]
              tunnel: w1781 -> [w1809]
              tunnel: w1780 -> [w1808]
              tunnel: w1779 -> [w1819]
              tunnel: w1778 -> [w1818]
              tunnel: [w1813] -> w1775
              tunnel: w1777 -> [w1813]
              tunnel: [w1812] -> w1774
              tunnel: w1776 -> [w1812]
              tunnel: [w1809] -> w1767
              tunnel: [w1808] -> w1765
              tunnel: [w1807] -> w1758
              tunnel: w1757 -> [w1807]
              tunnel: [w1806] -> w1754
              tunnel: w1753 -> [w1806]
              tunnel: [w1827] -> w1773
              tunnel: w1775 -> [w1827]
              tunnel: [w1826] -> w1772
              tunnel: w1774 -> [w1826]
              tunnel: w1767 -> [w1825]
              tunnel: [w1825] -> w1766
              tunnel: w1765 -> [w1824]
              tunnel: [w1824] -> w1764
              tunnel: [w1823] -> w1759
              tunnel: w1758 -> [w1823]
              tunnel: [w1822] -> w1755
              tunnel: w1754 -> [w1822]
              tunnel: w1773 -> [w1841]
              tunnel: w1772 -> [w1831]
              tunnel: [w1840] -> w1763
              tunnel: w1766 -> [w1830]
              tunnel: w1764 -> [w1829]
              tunnel: [w1834] -> w1761
              tunnel: [w1833] -> w1760
              tunnel: w1759 -> [w1833]
              tunnel: [w1832] -> w1756
              tunnel: w1755 -> [w1832]
              tunnel: [w1831] -> w1752
              tunnel: [w1830] -> w1751
              tunnel: [w1829] -> w1750
              tunnel: w1763 -> [w1863]
              tunnel: [w1863] -> w1762
              tunnel: w1761 -> [w1859]
              tunnel: w1760 -> [w1853]
              tunnel: w1756 -> [w1852]
              tunnel: w1752 -> [w1857]
              tunnel: w1751 -> [w1851]
              tunnel: w1750 -> [w1850]
              tunnel: [w1868] -> w1771
              tunnel: w1762 -> [w1865]
              frame #0 {
                w1805 = ".Pos"
                n715 = call <userlib>:"Open TCP-IP.vi"("IP address"=w1785) -> ("error out"=w1790:errorcluster, "Connection ID"=w1792:T9)  [unwired: 5 in, 4 out]
                n716 = Concatenate Strings(w1797, w1805) -> (w1786:string)
                n717 = Concatenate Strings(w1796, w1805) -> (w1787:string)
                n718 = call <userlib>:"Single Axis Group Position Current Get.vi"("error in (no error)"=w1790, "SingleAxis Group  Name (250 c max)"=w1787, "connection ID in"=w1792) -> ("error out"=w1793:errorcluster, "XPS error out"=w1794:errorcluster, "Current Position (units)"=w1783:dbl, "connection ID out"=w1795:T9)  [unwired: 5 in]
                "Pre-Capture Axis 1" <- w1783
                n719 = call <userlib>:"Single Axis Group Position Current Get.vi"("error in (no error)"=w1793, "XPS error in (no error)"=w1794, "SingleAxis Group  Name (250 c max)"=w1786, "connection ID in"=w1795) -> ("error out"=w1789:errorcluster, "XPS error out"=w1788:errorcluster, "Current Position (units)"=w1784:dbl, "connection ID out"=w1791:T9)  [unwired: 4 in]
                "Pre-Capture Axis 2" <- w1784
                n720 = local read "Axis Initial Parameters"() -> (w1798:T1)
                n721 = call <userlib>:"Positioner SGamma Parameters Set.vi"("SGamma Parameters"=w1798, "error in (no error)"=w1789, "XPS error in (no error)"=w1788, "Positioner Name (250 c max)"=w1787, "connection ID in"=w1791) -> ("error out"=w1802:errorcluster, "XPS error out"=w1803:errorcluster, "connection ID out"=w1804:T9)  [unwired: 4 in]
                n722 = call <userlib>:"Positioner SGamma Parameters Set.vi"("SGamma Parameters"=w1798, "error in (no error)"=w1802, "XPS error in (no error)"=w1803, "Positioner Name (250 c max)"=w1786, "connection ID in"=w1804) -> ("error out"=w1800:errorcluster, "XPS error out"=w1799:errorcluster, "connection ID out"=w1801:T9)  [unwired: 4 in]
              }
              frame #1 {
                n723 = local read "Axis 1 Offset"() -> (w1811:dbl)
                n724 = local read "Axis 2 Offset"() -> (w1810:dbl)
                n725 = call <userlib>:"Single Axis Group Move Relative.vi"("Target Displacement (units)"=w1811, "error in (no error)"=w1819, "XPS error in (no error)"=w1818, "SingleAxis Group  Name (250 c max)"=w1809, "connection ID in"=w1821) -> ("error out"=w1816:errorcluster, "XPS error out"=w1817:errorcluster, "connection ID out"=w1820:T9)  [unwired: 4 in]
                n726 = call <userlib>:"Single Axis Group Move Relative.vi"("Target Displacement (units)"=w1810, "error in (no error)"=w1816, "XPS error in (no error)"=w1817, "SingleAxis Group  Name (250 c max)"=w1808, "connection ID in"=w1820) -> ("error out"=w1814:errorcluster, "connection ID out"=w1815:T9)  [unwired: 4 in, 1 out]
                n727 = call <userlib>:"Close TCP-IP.vi"("error in (no error)"=w1814, "connection ID in"=w1815) -> ()  [unwired: 9 in, 1 out]
              }
              frame #2 {
                n728 = Wait (ms)(milliseconds to wait=u32 1000) -> ()  [unwired: 1 out]
              }
              frame #3 {
                n729 = local read "Speed (µm/s)"() -> (w1845:i32)
                n730 = local read "Processi time (sec)"() -> (w1839:i32)
                n731 = local read "Laser on/off array"() -> (w1848:bool[][])
                n732 = local read "Commands array"() -> (w1849:string[][])
                n733 = local read "ROI Area \n(mm2)"() -> (w1837:dbl)
                n734 = local read "Laser Com Delay"() -> (w1836:i32)
                n735 = local read "VISA Laser port"() -> (w1835:string)
                n736 = Divide(x=w1845, y=1000) -> (x/y=w1842:dbl)
                n737 = call "Capture.vi"("Commands array"=w1849, "XPS_Address"=w1831, "VISA resource name"=w1835, "laser array index"=0, "Process time"=w1839, "Axis Speed"=w1842, "Laser on/off array"=w1848, "stop"=FALSE ("STOP CAPTURE"), "delay before read (ms)"=w1836, "Axis Initial Parameters"=w1841, "ROI Area \n(mm2)"=w1837, "Axis 2"=w1829, "Axis 1"=w1830, "OPO on?"=TRUE, "Acceleration (units/seconds²)"="Acceleration \n(mm/s²)") -> ("Elapsed time"=w1840:dbl, "XPS error out"=w1834:errorcluster)  [unwired: 2 in, 1 out]
              }
              frame #4 {
                n738 = call <userlib>:"Open TCP-IP.vi"("IP address"=w1857) -> ("error out"=w1856:errorcluster, "Connection ID"=w1858:T9)  [unwired: 5 in, 4 out]
                n739 = call <userlib>:"Single Axis Group Move Absolute.vi"("Target Position (units)"=w1852, "error in (no error)"=w1856, "XPS error in (no error)"=w1859, "SingleAxis Group  Name (250 c max)"=w1851, "connection ID in"=w1858) -> ("error out"=w1861:errorcluster, "XPS error out"=w1860:errorcluster, "connection ID out"=w1862:T9)  [unwired: 4 in]
                n740 = call <userlib>:"Single Axis Group Move Absolute.vi"("Target Position (units)"=w1853, "error in (no error)"=w1861, "XPS error in (no error)"=w1860, "SingleAxis Group  Name (250 c max)"=w1850, "connection ID in"=w1862) -> ("error out"=w1854:errorcluster, "connection ID out"=w1855:T9)  [unwired: 4 in, 1 out]
                n741 = call <userlib>:"Close TCP-IP.vi"("error in (no error)"=w1854, "connection ID in"=w1855) -> ()  [unwired: 9 in, 1 out]
              }
              frame #5 {
                n742 = Number To Decimal String(number=w1865) -> (decimal integer string=w1864:string)  [unwired: 1 in]
                n743 = Concatenate Strings("Capture completed in " ("StringOut"), w1864, " seconds" ("string")) -> (w1868:string)
              }
            }
          }
        }
      }
      event "Microscope/Capture \nstatus button": Value Change {
        w1888 = 47 ("y")
        w1901 = "Ready"
        n744 = event-data() -> ()  [unwired: 1 in, 6 out]
        n745 = call <userlib>:"Open TCP-IP.vi"("IP address"=w1871) -> ("error out"=w1904:errorcluster, "Connection ID"=w1905:T9)  [unwired: 8 in, 1 out]
        n746 = call <vilib>:"Simple Error Handler.vi"("error in (no error)"=w1904) -> ("error?"=w1902:bool, "error out"=w1903:errorcluster)  [unwired: 4 in, 3 out]
        n747 = case shown="False" w1902 {
          tunnel: w1905 -> [w1983 _]
          tunnel: [w1980 w1987] -> w1887
          tunnel: [w1979 w1987] -> w1886
          tunnel: w1881 -> [w1978 _]
          tunnel: w1882 -> [w1977 _]
          tunnel: [w1975 w1988] -> w1885
          tunnel: [w1974 w1988] -> w1884
          tunnel: w1903 -> [w1971 _]
          frame False {
            n748 = call "Get Stages Status.vi"("error in (no error)"=w1971, "Group Name (250 c max)"=w1978, "connection ID in"=w1983) -> ("error out"=w1984:errorcluster, "XPS error out"=w1985:errorcluster, "Group Status String"=w1980:string, "connection ID out"=w1986:T9, "Status"=w1974:i32)  [unwired: 4 in]
            n749 = call "Get Stages Status.vi"("error in (no error)"=w1984, "XPS error in (no error)"=w1985, "Group Name (250 c max)"=w1977, "connection ID in"=w1986) -> ("error out"=w1981:errorcluster, "XPS error out"=w1976:errorcluster, "Group Status String"=w1979:string, "connection ID out"=w1982:T9, "Status"=w1975:i32)  [unwired: 3 in]
            n750 = call <vilib>:"Simple Error Handler.vi"("error source (\" \")"="Axes check" ("error source (\" \")"), "error in (no error)"=w1976) -> ()  [unwired: 3 in, 5 out]
            n751 = call <userlib>:"Close TCP-IP.vi"("error in (no error)"=w1981, "connection ID in"=w1982) -> ("Error out"=w1972:errorcluster)  [unwired: 9 in]
            n752 = call <vilib>:"Simple Error Handler.vi"("error in (no error)"=w1972) -> ()  [unwired: 4 in, 5 out]
          }
          frame True {
            w1988 = 0
            w1987 = ""
          }
        }
        n753 = Equal?(x=w1885, y=w1888) -> (x = y?=w1892:bool)
        n754 = Equal?(x=w1888, y=w1884) -> (x = y?=w1891:bool)
        n755 = String Subset(string=w1887, offset (0)=0, length (rest)=5 ("length (rest)")) -> (substring=w1899:string)
        n756 = String Subset(string=w1886, offset (0)=0, length (rest)=5 ("length (rest)")) -> (substring=w1900:string)
        n757 = case shown="False" "Microscope/Capture \nstatus button" {
          tunnel: ["capture " "microscope "] -> w1875
          frame False {
          }
          frame True {
          }
        }
        n758 = Equal?(x=w1899, y=w1901) -> (x = y?=w1898:bool)
        n759 = Equal?(x=w1901, y=w1900) -> (x = y?=w1897:bool)
        n760 = And(x=w1892, y=w1891) -> (x .and. y?=w1883:bool)
        n761 = Not(x=w1883) -> (.not. x?=w1889:bool)
        n762 = And(x=w1898, y=w1897) -> (x .and. y?=w1890:bool)
        n763 = And(x=w1890, y=w1889) -> (x .and. y?=w1873:bool)
        n764 = Concatenate Strings("Do you want to move the axis to the " ("message"), w1875, "position?" ("string")) -> (w1874:string)
        n765 = Two Button Dialog(message=w1874, 1:"No" ("F button name (\"Cancel\")"), 2:"Yes" ("T button name (\"OK\")")) -> (T button?=w1870:bool)
        n766 = case shown="False" w1870 {
          tunnel: "Microscope/Capture \nstatus button" -> [w1906 _]
          frame False {
            n767 = Not(x=w1906) -> (.not. x?=w1907:bool)
            n768 = local write "Microscope/Capture \nstatus button"(w1907) -> ()
          }
          frame True {
          }
        }
        n769 = And(x=w1873, y=w1870) -> (x .and. y?=w1872:bool)
        n770 = case shown="True" w1872 {
          tunnel: "Microscope/Capture \nstatus button" -> [w1911 w1916]
          tunnel: w1883 -> [w1912 _]
          tunnel: w1882 -> [_ w1924]
          tunnel: w1881 -> [_ w1923]
          tunnel: [_ w1922] -> w1880
          tunnel: w1871 -> [_ w1915]
          frame False {
            n771 = Not(x=w1911) -> (.not. x?=w1910:bool)
            n772 = case shown="True" w1912 {
              frame False {
                n773 = One Button Dialog(message="Axes are not ready") -> ()  [unwired: 1 in, 1 out]
              }
              frame True {
                n774 = One Button Dialog(message="One or more axis are in jogging mode") -> ()  [unwired: 1 in, 1 out]
              }
            }
            n775 = local write "Microscope/Capture \nstatus button"(w1910) -> ()
          }
          frame True {
            n776 = flat-sequence {
              tunnel: [w1935] -> w1921
              tunnel: [w1934] -> w1920
              tunnel: [w1933] -> w1919
              tunnel: [w1932] -> w1918
              tunnel: [w1931] -> w1917
              tunnel: w1924 -> [w1930]
              tunnel: w1923 -> [w1929]
              tunnel: w1915 -> [w1928]
              tunnel: w1921 -> [w1956]
              tunnel: w1920 -> [w1947]
              tunnel: w1919 -> [w1948]
              tunnel: w1918 -> [w1954]
              tunnel: w1917 -> [w1953]
              tunnel: w1916 -> [w1942]
              tunnel: [w1968] -> w1922
              tunnel: w1916 -> [w1964]
              frame #0 {
                w1940 = ".Pos"
                n777 = local read "Axis Initial Parameters"() -> (w1927:T1)
                n778 = Bundle By Name(cluster=w1927, "Velocity (units/seconds)"=10.0) -> (w1925:T1)
                n779 = call <userlib>:"Open TCP-IP.vi"("IP address"=w1928) -> ("error out"=w1936:errorcluster, "Connection ID"=w1941:T9)  [unwired: 5 in, 4 out]
                n780 = Concatenate Strings(w1929, w1940) -> (w1934:string)
                n781 = call <userlib>:"Positioner SGamma Parameters Set.vi"("SGamma Parameters"=w1927, "error in (no error)"=w1936, "Positioner Name (250 c max)"=w1934, "connection ID in"=w1941) -> ("error out"=w1937:errorcluster, "XPS error out"=w1938:errorcluster, "connection ID out"=w1939:T9)  [unwired: 5 in]
                n782 = Concatenate Strings(w1930, w1940) -> (w1933:string)
                n783 = call <userlib>:"Positioner SGamma Parameters Set.vi"("SGamma Parameters"=w1925, "error in (no error)"=w1937, "XPS error in (no error)"=w1938, "Positioner Name (250 c max)"=w1933, "connection ID in"=w1939) -> ("error out"=w1932:errorcluster, "XPS error out"=w1931:errorcluster, "connection ID out"=w1935:T9)  [unwired: 4 in]
              }
              frame #1 {
                n784 = local read "X travel"() -> (w1946:dbl)
                n785 = local read "Y travel"() -> (w1945:dbl)
                n786 = case shown="False" w1942 {
                  tunnel: w1946 -> [w1958 w1962]
                  tunnel: w1945 -> [w1957 w1961]
                  tunnel: [w1957 w1960] -> w1944
                  tunnel: [w1958 w1959] -> w1943
                  frame False {
                  }
                  frame True {
                    n787 = Negate(x=w1962) -> (-x=w1959:dbl)
                    n788 = Negate(x=w1961) -> (-x=w1960:dbl)
                  }
                }
                n789 = call <userlib>:"Single Axis Group Move Relative.vi"("Target Displacement (units)"=w1944, "error in (no error)"=w1954, "XPS error in (no error)"=w1953, "SingleAxis Group  Name (250 c max)"=w1947, "connection ID in"=w1956) -> ("error out"=w1951:errorcluster, "XPS error out"=w1952:errorcluster, "connection ID out"=w1955:T9)  [unwired: 4 in]
                n790 = call <userlib>:"Single Axis Group Move Relative.vi"("Target Displacement (units)"=w1943, "error in (no error)"=w1951, "XPS error in (no error)"=w1952, "SingleAxis Group  Name (250 c max)"=w1948, "connection ID in"=w1955) -> ("error out"=w1949:errorcluster, "connection ID out"=w1950:T9)  [unwired: 4 in, 1 out]
                n791 = call <userlib>:"Close TCP-IP.vi"("error in (no error)"=w1949, "connection ID in"=w1950) -> ()  [unwired: 9 in, 1 out]
              }
              frame #2 {
                n792 = Wait (ms)(milliseconds to wait=u32 1000) -> ()  [unwired: 1 out]
              }
              frame #3 {
                n793 = case shown="True" w1964 {
                  tunnel: ["capture " ("string") "microscope " ("string")] -> w1965
                  frame False {
                  }
                  frame True {
                  }
                }
                n794 = Concatenate Strings("Stages translated to the " ("StringOut"), w1965, "position." ("string")) -> (w1968:string)
              }
            }
          }
        }
      }
    }
    n795 = Get Date/Time In Seconds() -> (seconds since 1Jan1904=w816:timestamp)
    n796 = Format Date/Time String(time format string (%c)="%m/%d/%y - %I:%M %p  ", seconds (now)=w816) -> (date/time string=w815:string)  [unwired: 1 in]
    n797 = Empty String/Path?(string/path=w812) -> (empty?=w814:bool)
    n798 = Concatenate Strings(w815, w812, "\r") -> (w813:string)
    n799 = case shown="False" w814 {
      tunnel: w813 -> [w822 _]
      frame False {
        n800 = invoke on="Log" class="Str" method="Append String"("string"=w822) -> (error out=w821:errorcluster)  [unwired: 3 in, 3 out]
        n801 = property on="Log" class="Str"(error in=w821, "Text.Scroll Position"=u32 500000) -> ()  [unwired: 1 in, 2 out]
      }
      frame True {
      }
    }
  }
  n802 = control-ref of="Init Camera"() -> (w74:refnum<vi>)
  n803 = control-ref of="Stop Live"() -> (w67:refnum<vi>)
  n804 = property class="Bool"(reference=w67, "Disabled"=u8 2 ("Deaktiviert")) -> (reference out=w58:refnum<vi>, error out=w57:errorcluster)  [unwired: 1 in]
  n805 = property class="Bool"(reference=w74, "Disabled"=u8 0 ("Deaktiviert")) -> (reference out=w62:refnum<vi>, error out=w61:errorcluster)  [unwired: 1 in]
  n806 = Close Reference(reference=w58, error in (no error)=w57) -> ()  [unwired: 1 out]
  n807 = Close Reference(reference=w62, error in (no error)=w61) -> ()  [unwired: 1 out]
  n808 = control-ref of="Load Parameter"() -> (w68:refnum<vi>)
  n809 = control-ref of="Start Live"() -> (w71:refnum<vi>)
  n810 = property class="Bool"(reference=w71, "Disabled"=u8 2 ("Deaktiviert")) -> (reference out=w60:refnum<vi>, error out=w59:errorcluster)  [unwired: 1 in]
  n811 = property class="Bool"(reference=w68, "Disabled"=u8 2 ("Deaktiviert")) -> (reference out=w56:refnum<vi>, error out=w55:errorcluster)  [unwired: 1 in]
  n812 = Close Reference(reference=w60, error in (no error)=w59) -> ()  [unwired: 1 out]
  n813 = Close Reference(reference=w56, error in (no error)=w55) -> ()  [unwired: 1 out]
